vi "运维调试_质控单元.vi"() -> ()   [LabVIEW 2016, in "质控单元.lvlib"]
uses:
  <vilib>/Utility/miscctls.llb/LVPointTypeDef.ctl
  <vilib>/Utility/config.llb/Read Key (I32).vi
  <vilib>/Utility/config.llb/Read Key (Boolean).vi
  <vilib>/Utility/config.llb/Read Key (U32).vi
  <vilib>/Utility/config.llb/Write Key (I32).vi
  <vilib>/Utility/config.llb/Write Key (Boolean).vi
  <vilib>/Utility/config.llb/NI_LVConfig.lvlib
panel:
  out "CODCr状态簇":T1
  out "CODMn状态簇":T1
  out "总氮状态簇":T1
  out "总磷状态簇":T1
  out "氨氮状态簇":T1
  out "总氮柱塞泵故障报警":bool
  out "CODCr柱塞泵故障报警":bool
  out "CODMn柱塞泵故障报警":bool
  out "总磷柱塞泵故障报警":bool
  out "氨氮柱塞泵故障报警":bool
  out "总氮传感器故障报警":bool
  out "总氮传感器状态":bool
  out "总氮流程中断报警":bool
  out "总磷通讯":bool
  out "CODCr质控流程中":bool
  out "CODMn质控流程中":bool
  out "总氮质控流程中":bool caption="总磷质控流程中"
  out "总磷质控流程中":bool caption="总氮质控流程中"
  out "氨氮质控流程中":bool
  out "CODCr通讯":bool
  out "CODMn通讯":bool
  out "总氮通讯":bool
  out "氨氮通讯":bool
  out "CODCr传感器状态":bool
  out "CODCr传感器故障报警":bool
  out "CODMn传感器故障报警":bool
  out "总磷传感器故障报警":bool
  out "氨氮传感器故障报警":bool
  out "CODMn传感器状态":bool
  out "总磷传感器状态":bool
  out "氨氮传感器状态":bool
  out "CODCr流程中断报警":bool
  out "总磷流程中断报警":bool
  out "CODMn流程中断报警":bool
  out "氨氮流程中断报警":bool
  in  "总氮模块选择":bool
  in  "释放串口":bool
  in  "打开串口":bool
  in  "柱塞泵调试":bool
  in  "手动调试":bool
  in  "报警清除":bool
  in  "查看":bool
  in  "停止测量":bool
  in  "加标回收":bool
  in  "平行样测试":bool
  in  "CODCr量程选择":enum32{"H", "L", "AUTO"}(ring)
  in  "CODCr选择":bool
  out "CODCr加标回收率":dbl caption="加标回收率" format="%.2f"
  out "CODCr加标体积":dbl caption="加标体积" format="%.3f"
  out "CODCr母液浓度":dbl caption="加标母液浓度" format="%.2f"
  out "CODCr加标水杯定容体积":dbl caption="加标水杯定容体积" format="%.2f"
  out "CODCr加标后水样浓度":dbl caption="加标后水样浓度" format="%.2f"
  out "CODCr加标前水样浓度":dbl caption="加标前水样浓度" format="%.2f"
  out "CODCr检出限":dbl caption="检出限" format="%.2f"
  out "CODCr量程":dbl caption="量程" format="%.2f"
  out "CODCr状态":u16(ring) caption="状态" items=["待机", "润洗", "进样", "进样完成", "柱塞泵加标", "等待取液", "排液"]
  out "质控流程中":bool
  in  "CODMn量程选择":enum32{"H", "L", "AUTO"}(ring)
  in  "总磷量程选择":enum32{"H", "L", "AUTO"}(ring)=enum."AUTO"
  in  "总氮量程选择":enum32{"H", "L", "AUTO"}(ring)=enum."AUTO"
  in  "氨氮量程选择":enum32{"H", "L", "AUTO"}(ring)=enum."AUTO"
  in  "CODMn选择":bool
  in  "总磷模块选择":bool
  in  "氨氮模块":bool
  in  "背隙补偿步数 3":i32 min=0 max=2000
  in  "背隙补偿步数 2":i32 min=0 max=2000
  in  "背隙补偿步数":i32 min=0 max=2000
  out "总氮加标回收率":dbl caption="加标回收率" format="%.2f"
  out "总氮加标体积":dbl caption="加标体积" format="%.3f"
  out "总氮母液浓度":dbl caption="加标母液浓度" format="%.3f"
  out "总氮加标水杯定容体积":dbl caption="加标水杯定容体积" format="%.2f"
  out "总氮加标后水样浓度":dbl caption="加标后水样浓度" format="%.3f"
  out "总氮加标前水样浓度":dbl caption="加标前水样浓度" format="%.3f"
  out "总氮检出限":dbl caption="检出限" format="%.3f"
  out "总氮量程":dbl caption="量程" format="%.2f"
  out "总氮状态":u16(ring) caption="状态" items=["待机", "润洗", "进样", "进样完成", "柱塞泵加标", "等待取液", "排液"]
  in  "返回":bool
  out "COD平行样测完标志":bool
  out "氨氮总磷平行样测完标志":bool
  out "COD加标回收率":dbl caption="加标回收率" format="%.2f"
  out "COD加标体积":dbl caption="加标体积" format="%.3f"
  out "COD母液浓度":dbl caption="加标母液浓度" format="%.2f"
  out "COD加标水杯定容体积":dbl caption="加标水杯定容体积" format="%.2f"
  out "COD加标后水样浓度":dbl caption="加标后水样浓度" format="%.2f"
  out "COD加标前水样浓度":dbl caption="加标前水样浓度" format="%.2f"
  out "COD检出限":dbl caption="检出限" format="%.2f"
  out "COD量程":dbl caption="量程" format="%.2f"
  out "CODMn状态":u16(ring) caption="状态" items=["待机", "润洗", "进样", "进样完成", "柱塞泵加标", "等待取液", "排液"]
  out "总磷加标回收率":dbl caption="加标回收率" format="%.2f"
  out "总磷加标体积":dbl caption="加标体积" format="%.3f"
  out "总磷母液浓度":dbl caption="加标母液浓度" format="%.3f"
  out "总磷加标水杯定容体积":dbl caption="加标水杯定容体积" format="%.2f"
  out "总磷加标后水样浓度":dbl caption="加标后水样浓度" format="%.3f"
  out "总磷加标前水样浓度":dbl caption="加标前水样浓度" format="%.3f"
  out "总磷检出限":dbl caption="检出限" format="%.3f"
  out "总磷量程":dbl caption="量程" format="%.2f"
  out "总磷状态":u16(ring) caption="状态" items=["待机", "润洗", "进样", "进样完成", "柱塞泵加标", "等待取液", "排液"]
  out "氨氮加标回收率":dbl caption="加标回收率" format="%.2f"
  out "氨氮加标体积":dbl caption="加标体积" format="%.3f"
  out "氨氮母液浓度":dbl caption="加标母液浓度" format="%.3f"
  out "氨氮加标水杯定容体积":dbl caption="加标水杯定容体积" format="%.2f"
  out "氨氮加标后水样浓度":dbl caption="加标后水样浓度" format="%.3f"
  out "氨氮加标前水样浓度":dbl caption="加标前水样浓度" format="%.3f"
  out "氨氮检出限":dbl caption="检出限" format="%.3f"
  out "氨氮量程":dbl caption="量程" format="%.2f"
  out "氨氮状态":u16(ring) caption="状态" items=["待机", "润洗", "进样", "进样完成", "柱塞泵加标", "等待取液", "排液"]
  # "氨氮质控参数"
  # "状态显示区"
  # "参数配置区"
  # "2000步等于1mL\n100步等于0.05mL\n20步等于0.01mL\n2步等于0.001mL\n（初始默认100步）"
  # "柱塞泵调试区"
  # "CODCr质控参数"
  # "%"
  # "mL"
  # "mg/L"
  # "mL"
  # "mg/L"
  # "mg/L"
  # "mg/L"
  # "mg/L"
  # "总氮质控参数"
  # "%"
  # "mL"
  # "mg/L"
  # "mL"
  # "mg/L"
  # "mg/L"
  # "mg/L"
  # "mg/L"
  # "CODMn质控参数"
  # "%"
  # "mL"
  # "mg/L"
  # "mL"
  # "mg/L"
  # "mg/L"
  # "mg/L"
  # "mg/L"
  # "总磷质控参数"
  # "%"
  # "mL"
  # "mg/L"
  # "mL"
  # "mg/L"
  # "mg/L"
  # "mg/L"
  # "mg/L"
  # "%"
  # "mL"
  # "mg/L"
  # "mL"
  # "mg/L"
  # "mg/L"
  # "mg/L"
  # "mg/L"
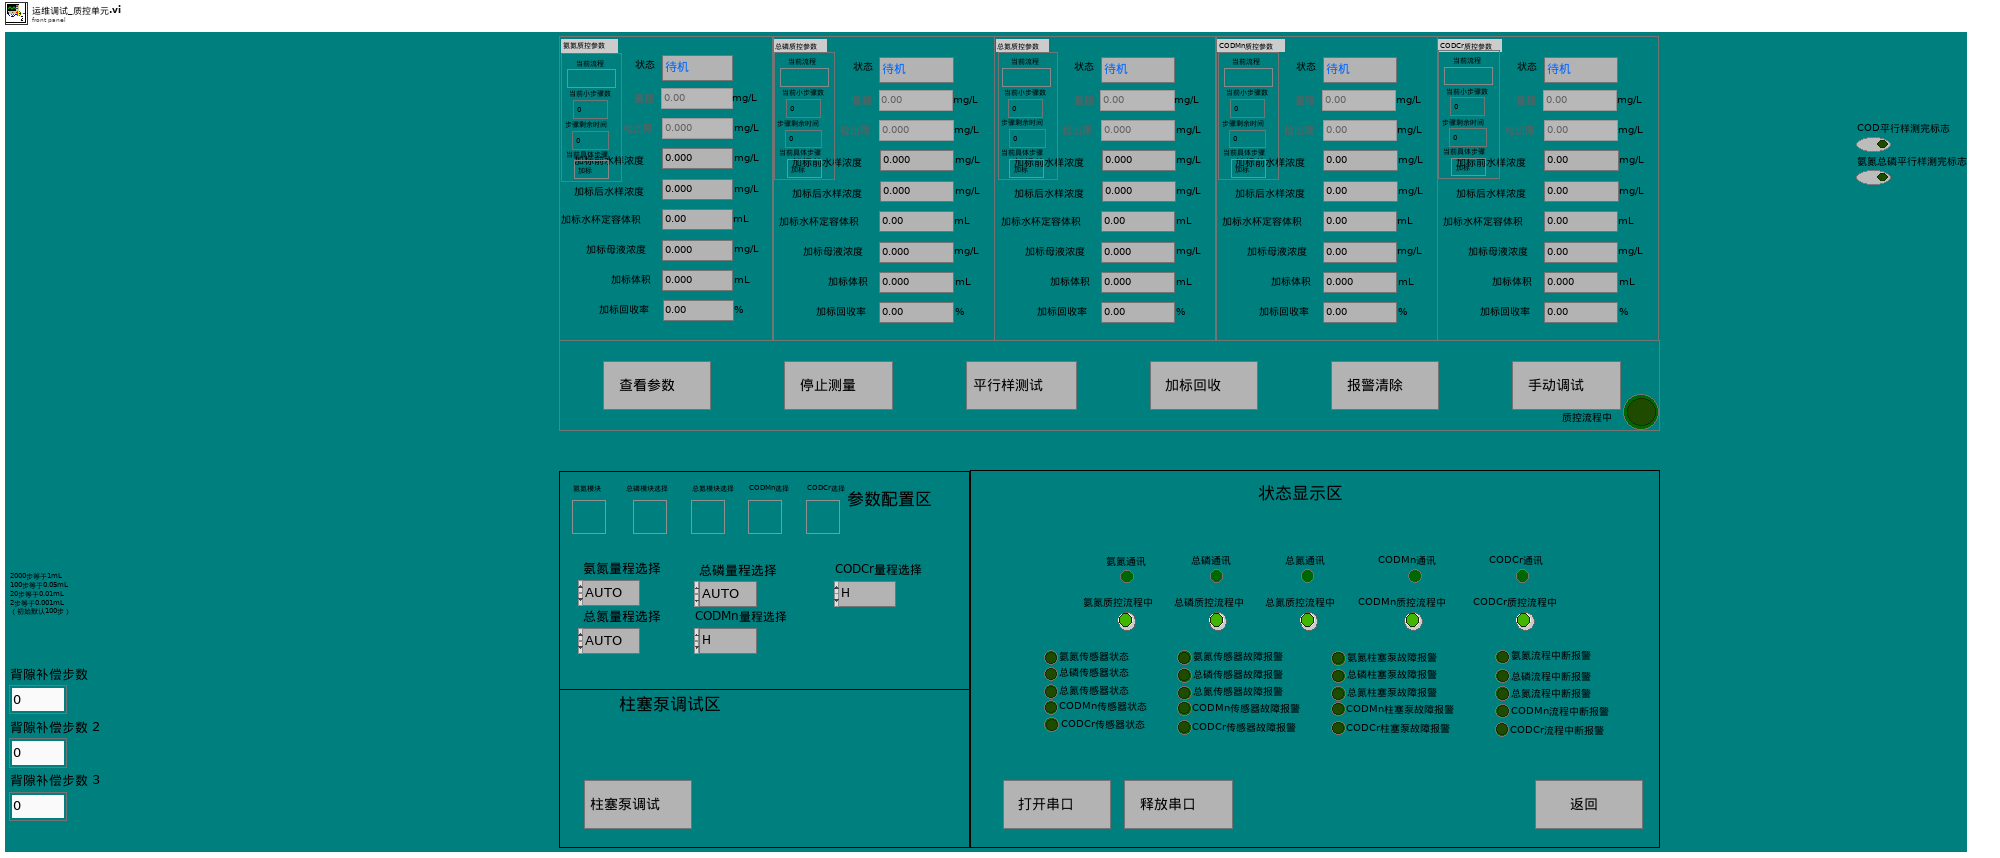
[diagram p1: front panel]
types:
  T1 = cluster{"步骤剩余时间":u16, "当前具体步骤":enum16{"加标", "进样", "排液", "搅拌", "定量"}, " 当前流程":enum16{"", "水样流程", "加标流程", "排液流程"}, "当前小步骤数":i8}
  T2 = typedef "LVPointTypeDef.ctl" = cluster{"Horizontal":i16, "Vertical":i16}
  T3 = typedef "NI_LVConfig.lvlib/Config Data RefNum.ctl" = refnum<k1>
  T4 = cluster{"量程":dbl, "检出限":dbl, "加标前水样浓度":dbl, "加标后水样浓度":dbl, "加标水杯定容体积":dbl, "加标母液浓度":dbl, "加标体积":dbl, "加标回收率":dbl}
  T5 = enum8{"Enabled", "Disabled", "Disabled and Grayed Out"}
  T6 = cluster{"是否启用仪器":bool, "CODMn":cluster{"启动测量模式":cluster{"测量模式":enum16{"水样测量", "标样核查", "加标回收", "平行样", "校零", "校标"}}, "确定按钮":bool}, "启动模块":cluster{"氨氮":bool, "总磷":bool, "总氮":bool, "CODMn":bool, "CODCr":bool}, "常规启动":bool, "直接启动":bool}
  T7 = cluster{"参数启用":cluster{"CODMn":bool, "总磷":bool, "总氮":bool, "氨氮":bool, "CODcr":bool}, "采配水是否启动":bool}
  T8 = cluster{"命令":string, cluster{"starting address":u16, "holding register value":u16}}
  T9 = cluster{"氨氮":bool, "总磷":bool, "总氮":bool, "CODMn":bool, "CODCr":bool}
  T10 = enum32{"Bad", "Idle", "Run top level", "Running"}
  T11 = cluster{"CODMn":bool, "总磷":bool, "总氮":bool, "氨氮":bool, "CODCr":bool}
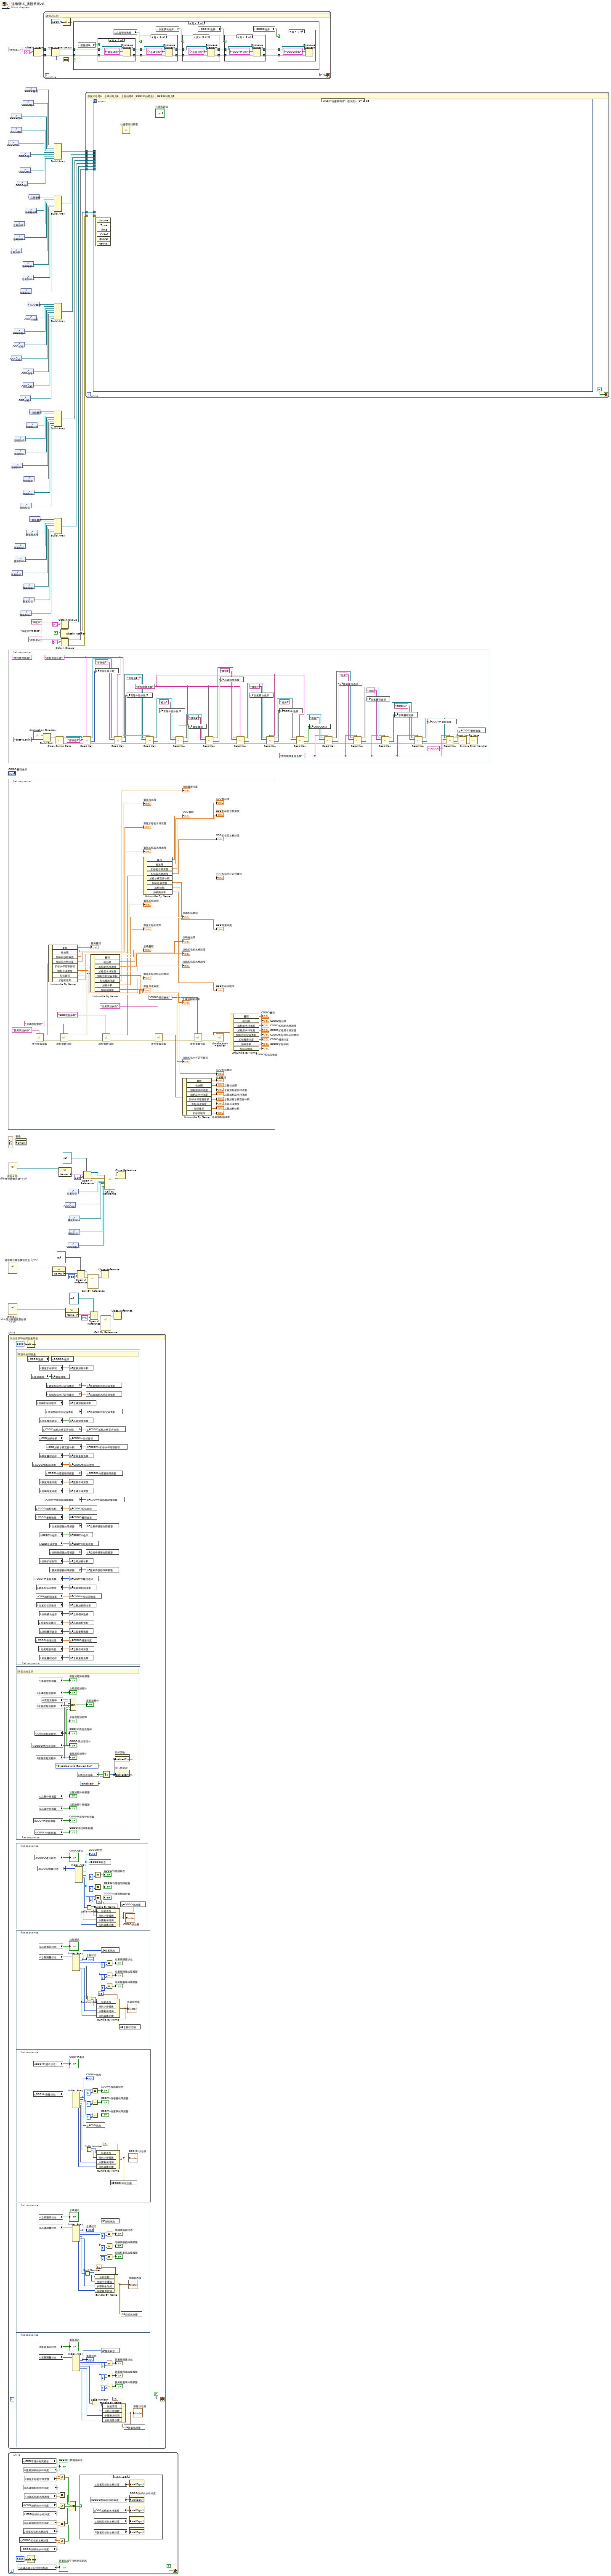
[diagram p0: block diagram]
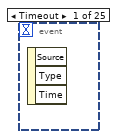
[diagram p9: hidden frame]
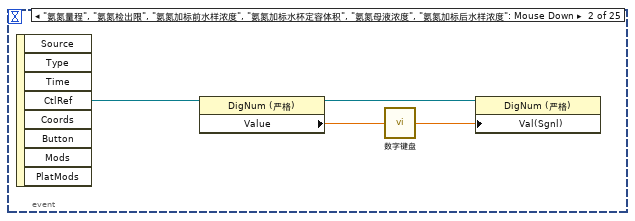
[diagram p10: hidden frame]
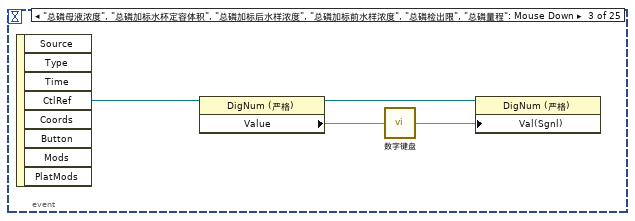
[diagram p11: hidden frame]
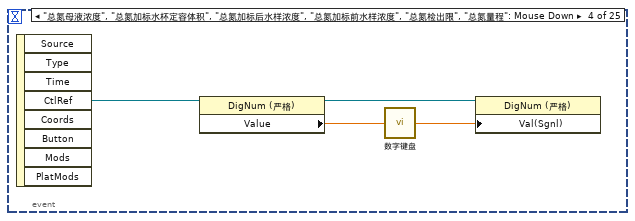
[diagram p12: hidden frame]
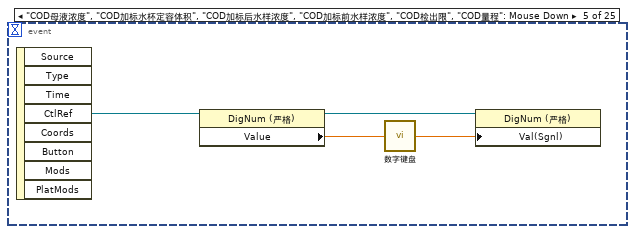
[diagram p13: hidden frame]
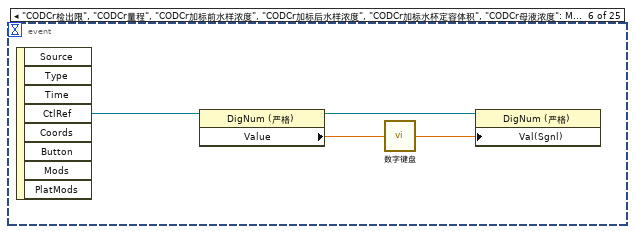
[diagram p14: hidden frame]
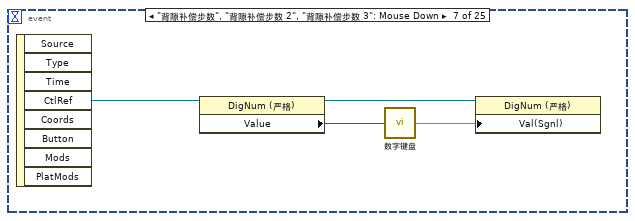
[diagram p15: hidden frame]
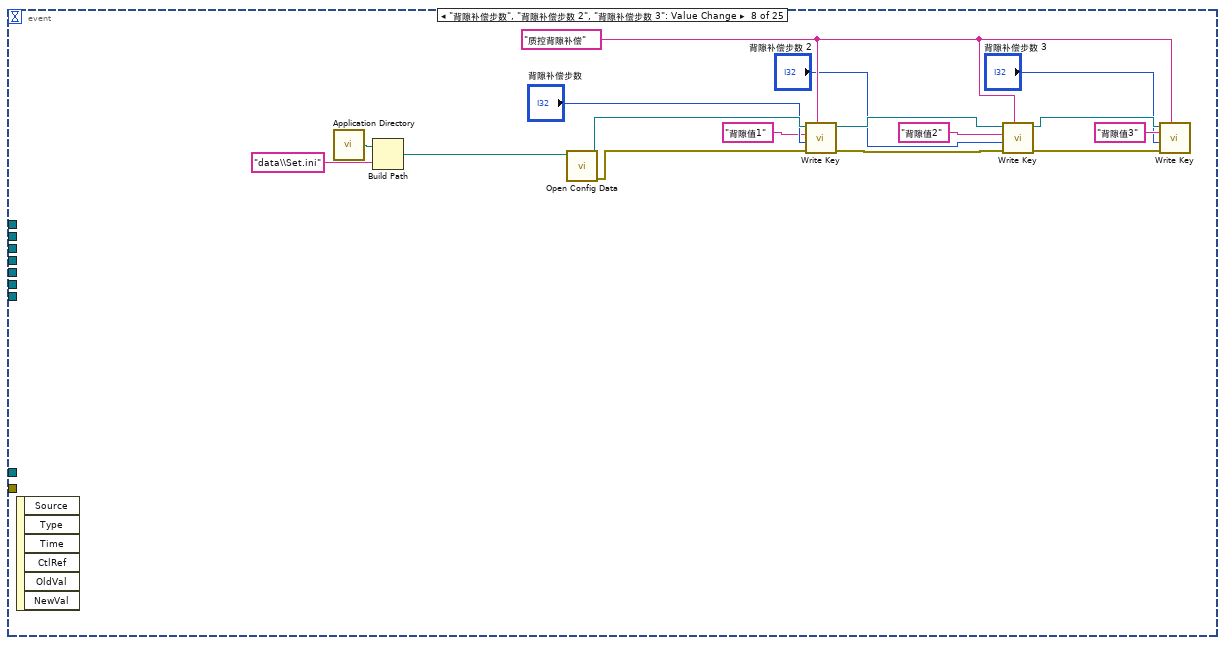
[diagram p16: hidden frame]
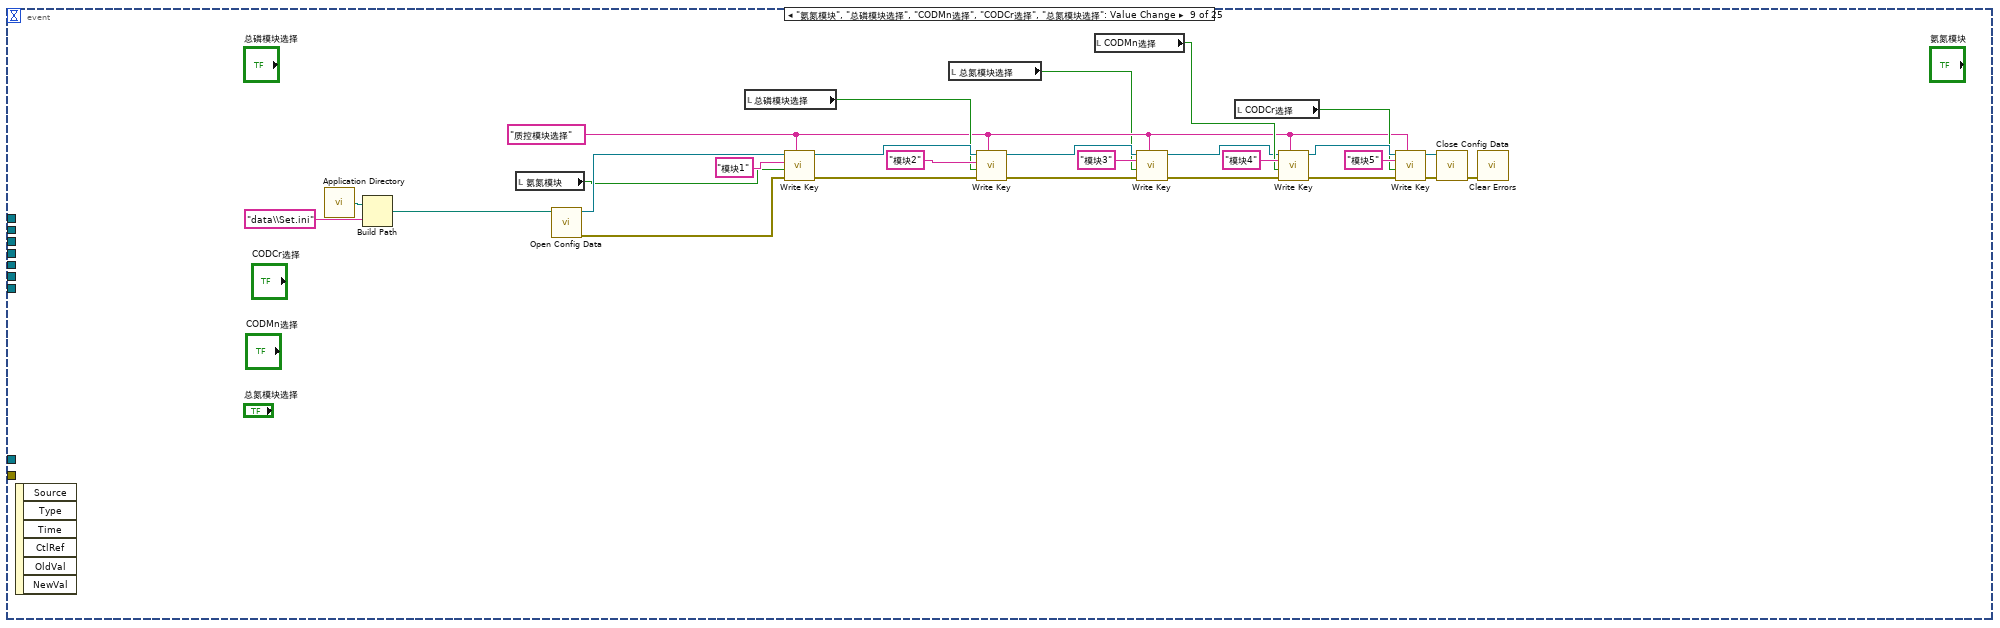
[diagram p17: hidden frame]
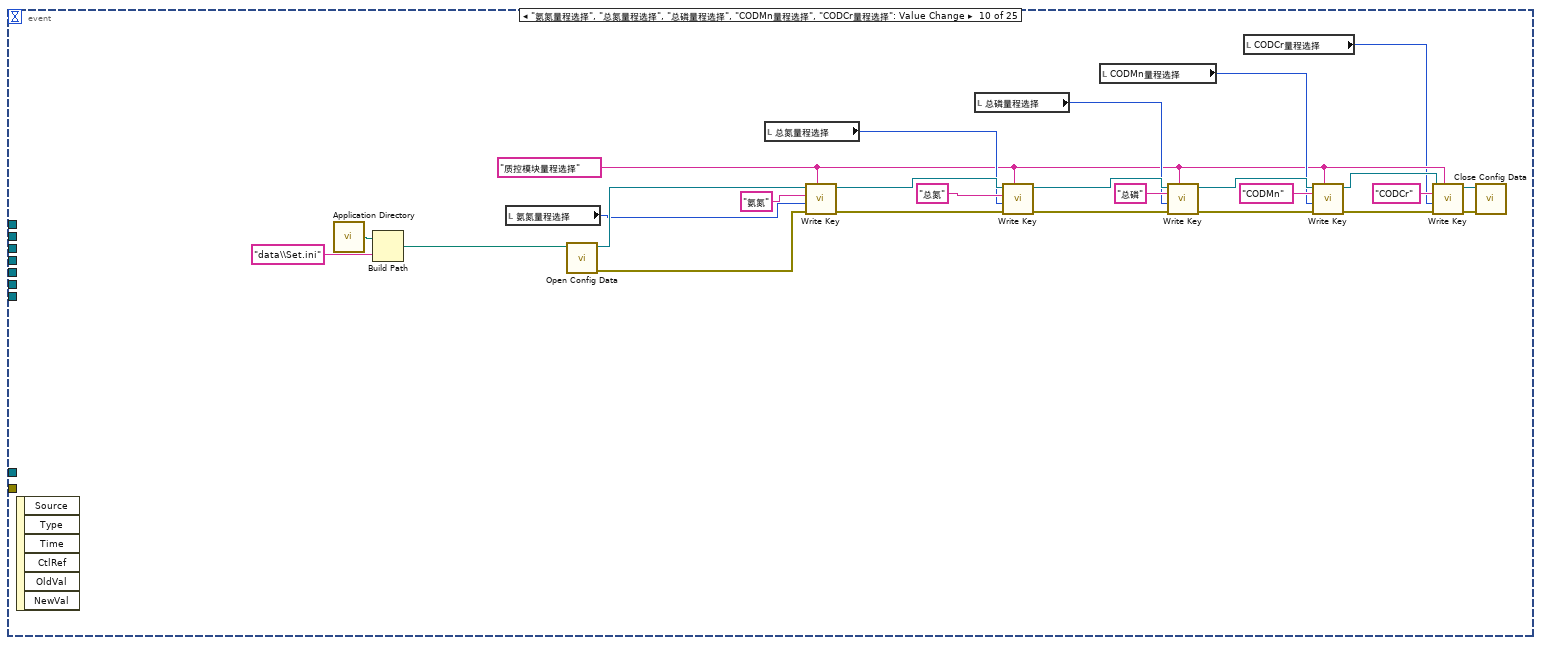
[diagram p18: hidden frame]
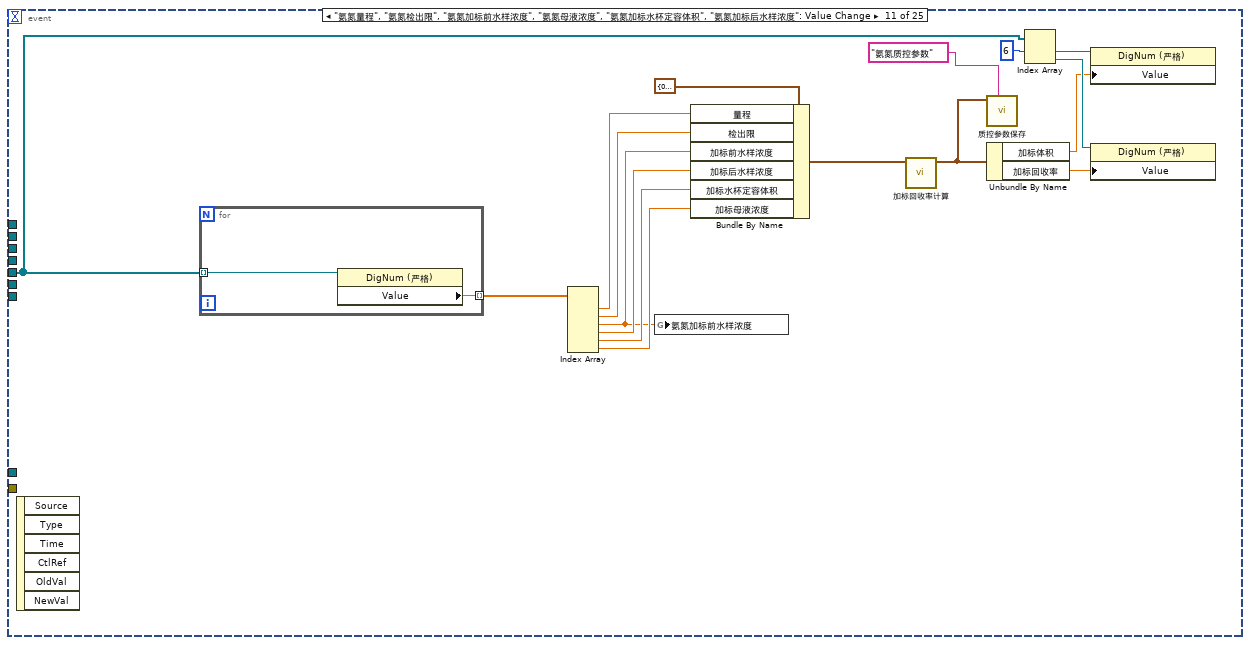
[diagram p19: hidden frame]
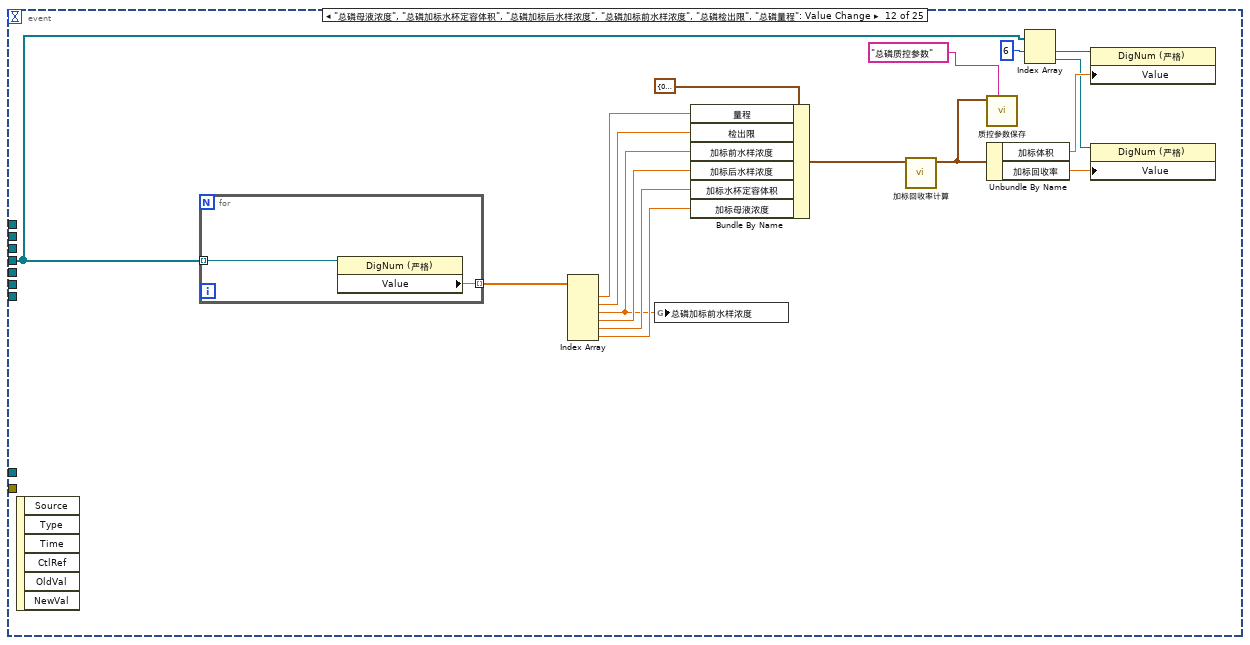
[diagram p20: hidden frame]
diagram:
  n1 = control-ref of="CODCr加标水杯定容体积"() -> (w42:refnum<vi>)
  n2 = flat-sequence {
    frame #0 {
      w110 = "质控模块量程选择" ("section")
      w91 = "质控模块选择" ("section")
      (unwired) "质控线性参数" ("section")
      w144 = "质控背隙补偿" ("section")
      n3 = call <vilib>:"Application Directory.vi"() -> ("Application Directory"=w150:path)
      n4 = Build Path(base path=w150, name or relative path="data\\Set.ini" ("名称或相对路径")) -> (appended path=w148:path)
      n5 = call <vilib>:"Open Config Data.vi"("configuration file path"=w148) -> ("error out"=w146:errorcluster, "refnum"=w147:T3)  [unwired: 8 in, 1 out]
      n6 = call-poly <vilib>:"Read Key.vi"("section"=w144, "error in (no error)"=w146, "key"="背隙值1", "refnum"=w147) -> ("error out"=w141:errorcluster, "value"=w136:i32, "refnum out"=w143:T3)  [unwired: 4 in, 1 out]
      n7 = local write "背隙补偿步数"(w136) -> ()
      n8 = call-poly <vilib>:"Read Key.vi"("section"=w144, "error in (no error)"=w141, "key"="背隙值2", "refnum"=w143) -> ("error out"=w139:errorcluster, "value"=w137:i32, "refnum out"=w140:T3)  [unwired: 4 in, 1 out]
      n9 = local write "背隙补偿步数 2"(w137) -> ()
      n10 = call-poly <vilib>:"Read Key.vi"("section"=w144, "error in (no error)"=w139, "key"="背隙值3", "refnum"=w140) -> ("error out"=w98:errorcluster, "value"=w135:i32, "refnum out"=w99:T3)  [unwired: 4 in, 1 out]
      n11 = local write "背隙补偿步数 3"(w135) -> ()
      n12 = call-poly <vilib>:"Read Key.vi"("section"=w91, "error in (no error)"=w98, "key"="模块1" ("section"), "refnum"=w99) -> ("error out"=w133:errorcluster, "value"=w127:bool, "refnum out"=w134:T3)  [unwired: 4 in, 1 out]
      n13 = local write "氨氮模块"(w127) -> ()
      n14 = call-poly <vilib>:"Read Key.vi"("section"=w91, "error in (no error)"=w133, "key"="模块2" ("section"), "refnum"=w134) -> ("error out"=w95:errorcluster, "value"=w128:bool, "refnum out"=w96:T3)  [unwired: 4 in, 1 out]
      n15 = local write "总磷模块选择"(w128) -> ()
      n16 = call-poly <vilib>:"Read Key.vi"("section"=w91, "error in (no error)"=w95, "key"="模块3" ("section"), "refnum"=w96) -> ("error out"=w93:errorcluster, "value"=w92:bool, "refnum out"=w94:T3)  [unwired: 4 in, 1 out]
      n17 = local write "总氮模块选择"(w92) -> ()
      n18 = call-poly <vilib>:"Read Key.vi"("section"=w91, "error in (no error)"=w93, "key"="模块4" ("section"), "refnum"=w94) -> ("error out"=w104:errorcluster, "value"=w129:bool, "refnum out"=w105:T3)  [unwired: 4 in, 1 out]
      n19 = local write "CODMn选择"(w129) -> ()
      n20 = call-poly <vilib>:"Read Key.vi"("section"=w91, "error in (no error)"=w104, "key"="模块5", "refnum"=w105) -> ("error out"=w101:errorcluster, "value"=w100:bool, "refnum out"=w102:T3)  [unwired: 4 in, 1 out]
      n21 = local write "CODCr选择"(w100) -> ()
      n22 = call-poly <vilib>:"Read Key.vi"("section"=w110, "error in (no error)"=w101, "key"="氨氮" ("section"), "refnum"=w102) -> ("error out"=w125:errorcluster, "value"=w116:u32, "refnum out"=w126:T3)  [unwired: 4 in, 1 out]
      n23 = local write "氨氮量程选择"(w116) -> ()
      n24 = call-poly <vilib>:"Read Key.vi"("section"=w110, "error in (no error)"=w125, "key"="总氮" ("section"), "refnum"=w126) -> ("error out"=w123:errorcluster, "value"=w115:u32, "refnum out"=w124:T3)  [unwired: 4 in, 1 out]
      n25 = local write "总氮量程选择"(w115) -> ()
      n26 = call-poly <vilib>:"Read Key.vi"("section"=w110, "error in (no error)"=w123, "key"="总磷" ("section"), "refnum"=w124) -> ("error out"=w121:errorcluster, "value"=w114:u32, "refnum out"=w122:T3)  [unwired: 4 in, 1 out]
      n27 = local write "总磷量程选择"(w114) -> ()
      n28 = call-poly <vilib>:"Read Key.vi"("section"=w110, "error in (no error)"=w121, "key"="CODMn" ("section"), "refnum"=w122) -> ("error out"=w111:errorcluster, "value"=w113:u32, "refnum out"=w112:T3)  [unwired: 4 in, 1 out]
      n29 = local write "CODMn量程选择"(w113) -> ()
      n30 = call-poly <vilib>:"Read Key.vi"("section"=w110, "error in (no error)"=w111, "key"="CODCr" ("section"), "refnum"=w112) -> ("error out"=w107:errorcluster, "value"=w108:u32, "refnum out"=w106:T3)  [unwired: 4 in, 1 out]
      n31 = local write "CODCr量程选择"(w108) -> ()
      n32 = call <vilib>:"Close Config Data.vi"("error in (no error)"=w107, "refnum"=w106) -> ("error out"=w90:errorcluster)  [unwired: 8 in, 1 out]
      n33 = call <vilib>:"Simple Error Handler.vi"("error in (no error)"=w90) -> ()  [unwired: 4 in, 5 out]
    }
  }
  n34 = flat-sequence {
    frame #0 {
      n35 = call "质控参数读取.vi"("section"="氨氮质控参数") -> ("error out"=w185:errorcluster, "参数"=w204:T4)  [unwired: 9 in]
      n36 = Unbundle By Name(w204) -> ("量程"=→"氨氮量程":dbl, "检出限"=→"氨氮检出限":dbl, "加标前水样浓度"=→"氨氮加标前水样浓度":dbl, "加标后水样浓度"=→"氨氮加标后水样浓度":dbl, "加标水杯定容体积"=→"氨氮加标水杯定容体积":dbl, "加标母液浓度"=→"氨氮母液浓度":dbl, "加标体积"=→"氨氮加标体积":dbl, "加标回收率"=→"氨氮加标回收率":dbl)
      n37 = call "质控参数读取.vi"("section"="总磷质控参数", "error in (no error)"=w185) -> ("error out"=w182:errorcluster, "参数"=w194:T4)  [unwired: 8 in]
      n38 = Unbundle By Name(w194) -> ("量程"=→"总磷量程":dbl, "检出限"=→"总磷检出限":dbl, "加标前水样浓度"=→"总磷加标前水样浓度":dbl, "加标后水样浓度"=→"总磷加标后水样浓度":dbl, "加标水杯定容体积"=→"总磷加标水杯定容体积":dbl, "加标母液浓度"=→"总磷母液浓度":dbl, "加标体积"=→"总磷加标体积":dbl, "加标回收率"=→"总磷加标回收率":dbl)
      n39 = call "质控参数读取.vi"("section"="COD质控参数", "error in (no error)"=w182) -> ("error out"=w172:errorcluster, "参数"=w184:T4)  [unwired: 8 in]
      n40 = Unbundle By Name(w184) -> ("量程"=→"COD量程":dbl, "检出限"=→"COD检出限":dbl, "加标前水样浓度"=→"COD加标前水样浓度":dbl, "加标后水样浓度"=→"COD加标后水样浓度":dbl, "加标水杯定容体积"=→"COD加标水杯定容体积":dbl, "加标母液浓度"=→"COD母液浓度":dbl, "加标体积"=→"COD加标体积":dbl, "加标回收率"=→"COD加标回收率":dbl)
      n41 = call "质控参数读取.vi"("section"="总氮质控参数", "error in (no error)"=w172) -> ("error out"=w160:errorcluster, "参数"=w171:T4)  [unwired: 8 in]
      n42 = Unbundle By Name(w171) -> ("量程"=→"总氮量程":dbl, "检出限"=→"总氮检出限":dbl, "加标前水样浓度"=→"总氮加标前水样浓度":dbl, "加标后水样浓度"=→"总氮加标后水样浓度":dbl, "加标水杯定容体积"=→"总氮加标水杯定容体积":dbl, "加标母液浓度"=→"总氮母液浓度":dbl, "加标体积"=→"总氮加标体积":dbl, "加标回收率"=→"总氮加标回收率":dbl)
      n43 = call "质控参数读取.vi"("section"="CODCr质控参数", "error in (no error)"=w160) -> ("error out"=w151:errorcluster, "参数"=w161:T4)  [unwired: 8 in]
      n44 = call <vilib>:"Simple Error Handler.vi"("error in (no error)"=w151) -> ()  [unwired: 4 in, 5 out]
      n45 = Unbundle By Name(w161) -> ("量程"=→"CODCr量程":dbl, "检出限"=→"CODCr检出限":dbl, "加标前水样浓度"=→"CODCr加标前水样浓度":dbl, "加标后水样浓度"=→"CODCr加标后水样浓度":dbl, "加标水杯定容体积"=→"CODCr加标水杯定容体积":dbl, "加标母液浓度"=→"CODCr母液浓度":dbl, "加标体积"=→"CODCr加标体积":dbl, "加标回收率"=→"CODCr加标回收率":dbl)
    }
  }
  n46 = vi-ref "质控单元.lvlib:质控数据存储(子VI).vi"() -> (w17:refnum<vi>)
  n47 = vi-ref "通信并与其他模块交互 (子VI).vi"() -> (w30:refnum<vi>)
  n48 = vi-ref "质控单元.lvlib:质控报警信息存储 (子VI).vi"() -> (w25:refnum<vi>)
  n49 = while {
    stop <- FALSE stop-if-true
    # "状态显示和全局变量赋值"
    n50 = flat-sequence {
      frame #0 {
        # "赋值给全局变量"
        n51 = local read "CODCr选择"() -> (w341:bool)
        n52 = local read "氨氮模块"() -> (w340:bool)
        n53 = local read "CODCr加标回收率"() -> (w323:dbl)
        n54 = local read "CODMn量程选择"() -> (w347:enum32{"H", "L", "AUTO"})
        n55 = local read "CODCr加标体积"() -> (w334:dbl)
        n56 = local read "CODCr量程选择"() -> (w348:enum32{"H", "L", "AUTO"})
        n57 = local read "CODCr母液浓度"() -> (w324:dbl)
        n58 = local read "COD加标回收率"() -> (w322:dbl)
        n59 = local read "总磷加标回收率"() -> (w320:dbl)
        n60 = local read "氨氮加标回收率"() -> (w319:dbl)
        n61 = local read "总氮加标回收率"() -> (w321:dbl)
        n62 = local read "总氮加标体积"() -> (w336:dbl)
        n63 = local read "总氮母液浓度"() -> (w326:dbl)
        n64 = local read "COD加标体积"() -> (w335:dbl)
        n65 = local read "COD母液浓度"() -> (w325:dbl)
        n66 = local read "氨氮加标体积"() -> (w338:dbl)
        n67 = local read "总氮模块选择"() -> (w343:bool)
        n68 = local read "氨氮量程选择"() -> (w346:enum32{"H", "L", "AUTO"})
        n69 = local read "氨氮母液浓度"() -> (w328:dbl)
        n70 = local read "总磷母液浓度"() -> (w327:dbl)
        n71 = local read "总磷加标体积"() -> (w337:dbl)
        n72 = local read "总磷模块选择"() -> (w339:bool)
        n73 = local read "总磷量程选择"() -> (w344:enum32{"H", "L", "AUTO"})
        n74 = local read "总氮量程选择"() -> (w345:enum32{"H", "L", "AUTO"})
        n75 = local read "CODMn选择"() -> (w342:bool)
        n76 = local read "CODCr加标水杯定容体积"() -> (w333:dbl)
        n77 = local read "CODMn传感器故障报警"() -> (w315:bool)
        n78 = local read "总氮加标水杯定容体积"() -> (w331:dbl)
        n79 = local read "CODCr传感器故障报警"() -> (w314:bool)
        n80 = local read "COD加标水杯定容体积"() -> (w332:dbl)
        n81 = local read "氨氮加标水杯定容体积"() -> (w329:dbl)
        n82 = local read "总磷加标水杯定容体积"() -> (w330:dbl)
        n83 = local read "总氮传感器故障报警"() -> (w316:bool)
        n84 = local read "总磷传感器故障报警"() -> (w317:bool)
        n85 = local read "氨氮传感器故障报警"() -> (w318:bool)
        n86 = global write "断电保存全局.vi" "CODCr选择"(w341) -> ()
        n87 = global write "断电保存全局.vi" "氨氮模块"(w340) -> ()
        n88 = global write "加标回收状态全局变量.vi" "氨氮加标体积"(w338) -> ()
        n89 = global write "加标回收状态全局变量.vi" "总磷加标回收率"(w320) -> ()
        n90 = global write "断电保存全局.vi" "总氮模块选择"(w343) -> ()
        n91 = global write "加标回收状态全局变量.vi" "CODMn加标体积"(w335) -> ()
        n92 = global write "断电保存全局.vi" "氨氮量程选择"(w346) -> ()
        n93 = global write "加标回收状态全局变量.vi" "CODCr加标回收率"(w323) -> ()
        n94 = global write "加标回收状态全局变量.vi" "氨氮母液浓度"(w328) -> ()
        n95 = global write "加标回收状态全局变量.vi" "总磷母液浓度"(w327) -> ()
        n96 = global write "加标回收状态全局变量.vi" "CODCr加标体积"(w334) -> ()
        n97 = global write "断电保存全局.vi" "CODCr量程选择"(w348) -> ()
        n98 = global write "断电保存全局.vi" "CODMn选择"(w342) -> ()
        n99 = global write "加标回收状态全局变量.vi" "CODMn母液浓度"(w325) -> ()
        n100 = global write "加标回收状态全局变量.vi" "总磷加标体积"(w337) -> ()
        n101 = global write "断电保存全局.vi" "CODMn量程选择"(w347) -> ()
        n102 = global write "加标回收状态全局变量.vi" "氨氮加标回收率"(w319) -> ()
        n103 = global write "加标回收状态全局变量.vi" "CODMn加标回收率"(w322) -> ()
        n104 = global write "加标回收状态全局变量.vi" "总氮加标回收率"(w321) -> ()
        n105 = global write "断电保存全局.vi" "总磷模块选择"(w339) -> ()
        n106 = global write "加标回收状态全局变量.vi" "总氮加标体积"(w336) -> ()
        n107 = global write "断电保存全局.vi" "总磷量程选择"(w344) -> ()
        n108 = global write "加标回收状态全局变量.vi" "CODCr母液浓度"(w324) -> ()
        n109 = global write "加标回收状态全局变量.vi" "总氮母液浓度"(w326) -> ()
        n110 = global write "断电保存全局.vi" "总氮量程选择"(w345) -> ()
        n111 = global write "加标回收状态全局变量.vi" "氨氮加标水杯定容体积"(w329) -> ()
        n112 = global write "加标回收状态全局变量.vi" "总磷加标水杯定容体积"(w330) -> ()
        n113 = global write "加标回收状态全局变量.vi" "总氮加标水杯定容体积"(w331) -> ()
        n114 = global write "加标回收状态全局变量.vi" "CODCr加标水杯定容体积"(w333) -> ()
        n115 = global write "加标回收状态全局变量.vi" "CODMn加标水杯定容体积"(w332) -> ()
        n116 = global write "质控中断报警全局.vi" "CODCr传感器故障报警"(w314) -> ()
        n117 = global write "质控中断报警全局.vi" "CODMn传感器故障报警"(w315) -> ()
        n118 = global write "质控中断报警全局.vi" "总氮传感器故障报警"(w316) -> ()
        n119 = global write "质控中断报警全局.vi" "总磷传感器故障报警"(w317) -> ()
        n120 = global write "质控中断报警全局.vi" "氨氮传感器故障报警"(w318) -> ()
      }
    }
    n121 = flat-sequence {
      frame #0 {
        # "界面状态显示"
        n122 = global read "质控测完标志全局 1.vi" "CODCr质控流程中"() -> (w304:bool)
        "CODCr质控流程中" <- w304
        n123 = global read "质控中断报警全局.vi" "CODMn中断报警"() -> (→"CODMn流程中断报警":bool)
        n124 = global read "质控测完标志全局 1.vi" "COD质控流程中"() -> (w303:bool)
        "CODMn质控流程中" <- w303
        n125 = global read "质控中断报警全局.vi" "CODCr中断报警"() -> (→"CODCr流程中断报警":bool)
        n126 = global read "质控测完标志全局 1.vi" "总磷质控流程中"() -> (w302:bool)
        "总磷质控流程中" <- w302
        n127 = global read "质控测完标志全局 1.vi" "总氮质控流程中"() -> (w305:bool)
        "总氮质控流程中" <- w305
        n128 = global read "质控测完标志全局 1.vi" "氨氮质控流程中"() -> (w301:bool)
        "氨氮质控流程中" <- w301
        n129 = global read "质控中断报警全局.vi" "氨氮中断报警"() -> (→"氨氮流程中断报警":bool)
        n130 = global read "质控中断报警全局.vi" "总氮中断报警"() -> (→"总氮流程中断报警":bool)
        n131 = global read "质控中断报警全局.vi" "总磷中断报警"() -> (→"总磷流程中断报警":bool)
        n132 = global read "质控测完标志全局 1.vi" "质控流程中"() -> (w299:bool)
        n133 = Compound Arithmetic op=OR ("复合运算")(w299, w301, w302, w305, w303, w304) -> (→"质控流程中":bool)
        n134 = global read "质控测完标志全局 1.vi" "质控流程中"() -> (w309:bool)
        n135 = Select(t=T5."Disabled and Grayed Out" ("禁用"), s=w309, f=T5."Enabled") -> (s? t:f=w298:T5)
        n136 = property on="加标回收" class="Bool"("DisabledEnum"=w298) -> ()  [unwired: 2 in, 2 out]
        n137 = property on="平行样测试" class="Bool"("DisabledEnum"=w298) -> ()  [unwired: 2 in, 2 out]
      }
    }
    n138 = flat-sequence {
      frame #0 {
        n139 = global read "质控内部交互全局.vi" "CODCr通讯状态"() -> (→"CODCr通讯":bool)
        n140 = global read "质控内部交互全局.vi" "CODCr测量状态"() -> (w242:u16[])
        n141 = Index Array(array=w242) -> (element #1=w243:u16, element #2=w238:u16, element #3=w234:u16, element #4=w232:u16, element #5=w229:u16, element #6=w228:u16)  [unwired: 6 in]
        "CODCr状态" <- w243
        n142 = Split Number(x=w232) -> (hi(x)=w231:u8, lo(x)=w230:u8)
        n143 = global write "加标回收状态全局变量.vi" "CODCr状态"(w243) -> ()
        n144 = Equal?(x=w238, y=u16 1) -> (x = y?=→"CODCr传感器状态":bool)
        n145 = Equal?(x=w234, y=u16 1) -> (x = y?=→"CODCr传感器故障报警":bool)
        n146 = Equal?(x=w234, y=u16 2) -> (x = y?=→"CODCr柱塞泵故障报警":bool)
        n147 = Bundle By Name(cluster=T1 {"步骤剩余时间"=0, "当前具体步骤"=enum."加标", " 当前流程"=enum."", "当前小步骤数"=0} ("氨氮状态簇"), "当前流程"=w231, "当前小步骤数"=w230, "步骤剩余时间"=w229, "当前具体步骤"=w228) -> (w226:T1)
        "CODCr状态簇" <- w226
        n148 = global write "加标回收状态全局变量.vi" "CODCr状态簇"(w226) -> ()
      }
    }
    n149 = flat-sequence {
      frame #0 {
        n150 = global read "质控内部交互全局.vi" "总氮通讯状态"() -> (→"总氮通讯":bool)
        n151 = global read "质控内部交互全局.vi" "总氮测量状态"() -> (w222:u16[])
        n152 = Index Array(array=w222) -> (element #1=w221:u16, element #2=w224:u16, element #3=w216:u16, element #4=w212:u16, element #5=w210:u16, element #6=w211:u16)  [unwired: 6 in]
        "总氮状态" <- w221
        n153 = Split Number(x=w212) -> (hi(x)=w214:u8, lo(x)=w213:u8)
        n154 = Bundle By Name(cluster=T1 {"步骤剩余时间"=0, "当前具体步骤"=enum."加标", " 当前流程"=enum."", "当前小步骤数"=0} ("氨氮状态簇"), "当前流程"=w214, "当前小步骤数"=w213, "步骤剩余时间"=w210, "当前具体步骤"=w211) -> (w208:T1)
        "总氮状态簇" <- w208
        n155 = global write "加标回收状态全局变量.vi" "总氮状态"(w221) -> ()
        n156 = Equal?(x=w224, y=u16 1) -> (x = y?=→"总氮传感器状态":bool)
        n157 = Equal?(x=w216, y=u16 1) -> (x = y?=→"总氮传感器故障报警":bool)
        n158 = Equal?(x=w216, y=u16 2) -> (x = y?=→"总氮柱塞泵故障报警":bool)
        n159 = global write "加标回收状态全局变量.vi" "总氮状态簇"(w208) -> ()
      }
    }
    n160 = flat-sequence {
      frame #0 {
        n161 = global read "质控内部交互全局.vi" "CODMn通讯状态"() -> (→"CODMn通讯":bool)
        n162 = global read "质控内部交互全局.vi" "CODMn测量状态"() -> (w258:u16[])
        n163 = Index Array(array=w258) -> (element #1=w261:u16, element #2=w259:u16, element #3=w252:u16, element #4=w248:u16, element #5=w246:u16, element #6=w247:u16)  [unwired: 6 in]
        "CODMn状态" <- w261
        n164 = Split Number(x=w248) -> (hi(x)=w250:u8, lo(x)=w249:u8)
        n165 = global write "加标回收状态全局变量.vi" "COD状态"(w261) -> ()
        n166 = Equal?(x=w259, y=u16 1) -> (x = y?=→"CODMn传感器状态":bool)
        n167 = Equal?(x=w252, y=u16 1) -> (x = y?=→"CODMn传感器故障报警":bool)
        n168 = Equal?(x=w252, y=u16 2) -> (x = y?=→"CODMn柱塞泵故障报警":bool)
        n169 = Bundle By Name(cluster=T1 {"步骤剩余时间"=0, "当前具体步骤"=enum."加标", " 当前流程"=enum."", "当前小步骤数"=0} ("氨氮状态簇"), "当前流程"=w250, "当前小步骤数"=w249, "步骤剩余时间"=w246, "当前具体步骤"=w247) -> (w244:T1)
        "CODMn状态簇" <- w244
        n170 = global write "加标回收状态全局变量.vi" "CODMn状态簇"(w244) -> ()
      }
    }
    n171 = flat-sequence {
      frame #0 {
        n172 = global read "质控内部交互全局.vi" "总磷通讯状态"() -> (→"总磷通讯":bool)
        n173 = global read "质控内部交互全局.vi" "总磷测量状态"() -> (w276:u16[])
        n174 = Index Array(array=w276) -> (element #1=w277:u16, element #2=w278:u16, element #3=w270:u16, element #4=w266:u16, element #5=w264:u16, element #6=w265:u16)  [unwired: 6 in]
        "总磷状态" <- w277
        n175 = Split Number(x=w266) -> (hi(x)=w268:u8, lo(x)=w267:u8)
        n176 = Bundle By Name(cluster=T1 {"步骤剩余时间"=0, "当前具体步骤"=enum."加标", " 当前流程"=enum."", "当前小步骤数"=0} ("氨氮状态簇"), "当前流程"=w268, "当前小步骤数"=w267, "步骤剩余时间"=w264, "当前具体步骤"=w265) -> (w262:T1)
        "总磷状态簇" <- w262
        n177 = global write "加标回收状态全局变量.vi" "总磷状态"(w277) -> ()
        n178 = Equal?(x=w278, y=u16 1) -> (x = y?=→"总磷传感器状态":bool)
        n179 = Equal?(x=w270, y=u16 1) -> (x = y?=→"总磷传感器故障报警":bool)
        n180 = Equal?(x=w270, y=u16 2) -> (x = y?=→"总磷柱塞泵故障报警":bool)
        n181 = global write "加标回收状态全局变量.vi" "总磷状态簇"(w262) -> ()
      }
    }
    n182 = flat-sequence {
      frame #0 {
        n183 = global read "质控内部交互全局.vi" "氨氮通讯状态"() -> (→"氨氮通讯":bool)
        n184 = global read "质控内部交互全局.vi" "氨氮测量状态"() -> (w294:u16[])
        n185 = Index Array(array=w294) -> (element #1=w295:u16, element #2=w297:u16, element #3=w288:u16, element #4=w284:u16, element #5=w282:u16, element #6=w283:u16)  [unwired: 6 in]
        "氨氮状态" <- w295
        n186 = Split Number(x=w284) -> (hi(x)=w286:u8, lo(x)=w285:u8)
        n187 = global write "加标回收状态全局变量.vi" "氨氮状态"(w295) -> ()
        n188 = Bundle By Name(cluster=T1 {"步骤剩余时间"=0, "当前具体步骤"=enum."加标", " 当前流程"=enum."", "当前小步骤数"=0} ("氨氮状态簇"), "当前流程"=w286, "当前小步骤数"=w285, "步骤剩余时间"=w282, "当前具体步骤"=w283) -> (w280:T1)
        "氨氮状态簇" <- w280
        n189 = Equal?(x=w297, y=u16 1) -> (x = y?=→"氨氮传感器状态":bool)
        n190 = Equal?(x=w288, y=u16 1) -> (x = y?=→"氨氮传感器故障报警":bool)
        n191 = Equal?(x=w288, y=u16 2) -> (x = y?=→"氨氮柱塞泵故障报警":bool)
        n192 = global write "加标回收状态全局变量.vi" "氨氮状态簇"(w280) -> ()
      }
    }
    n193 = Wait (ms)(milliseconds to wait=u32 1000 ("等待时间（毫秒）")) -> ()  [unwired: 1 out]
  }
  n194 = while {
    stop <- FALSE stop-if-true
    n195 = global read "质控测完标志全局 1.vi" "总磷总氮平行样测完标志"() -> (→"氨氮总磷平行样测完标志":bool)
    n196 = global read "水样浓度全局.vi" "CODCr加标前水样浓度"() -> (w351:dbl)
    n197 = local read "CODCr加标前水样浓度"() -> (w350:dbl)
    n198 = global read "质控测完标志全局 1.vi" "COD平行样测完标志"() -> (→"COD平行样测完标志":bool)
    n199 = global read "水样浓度全局.vi" "COD加标前水样浓度"() -> (w362:dbl)
    n200 = local read "总氮加标前水样浓度"() -> (w354:dbl)
    n201 = global read "水样浓度全局.vi" "氨氮加标前水样浓度"() -> (w366:dbl)
    n202 = global read "水样浓度全局.vi" "总磷加标前水样浓度"() -> (w364:dbl)
    n203 = local read "COD加标前水样浓度"() -> (w361:dbl)
    n204 = global read "水样浓度全局.vi" "总氮加标前水样浓度"() -> (w353:dbl)
    n205 = local read "氨氮加标前水样浓度"() -> (w365:dbl)
    n206 = local read "总磷加标前水样浓度"() -> (w363:dbl)
    n207 = Wait (ms)(milliseconds to wait=u32 1000 ("等待时间（毫秒）")) -> ()  [unwired: 1 out]
    n208 = Not Equal?(x=w366, y=w365) -> (x != y?=w360:bool)
    n209 = Not Equal?(x=w364, y=w363) -> (x != y?=w358:bool)
    n210 = Not Equal?(x=w362, y=w361) -> (x != y?=w357:bool)
    n211 = Not Equal?(x=w353, y=w354) -> (x != y?=w352:bool)
    n212 = Not Equal?(x=w351, y=w350) -> (x != y?=w349:bool)
    n213 = Compound Arithmetic op=OR ("复合运算")(w360, w358, w357, w352, w349) -> (w359:bool)
    n214 = case shown="真" w359 {
      frame False {
      }
      frame True {
        n215 = global read "水样浓度全局.vi" "CODCr加标前水样浓度"() -> (w369:dbl)
        n216 = global read "水样浓度全局.vi" "COD加标前水样浓度"() -> (w371:dbl)
        n217 = global read "水样浓度全局.vi" "总氮加标前水样浓度"() -> (w370:dbl)
        n218 = global read "水样浓度全局.vi" "总磷加标前水样浓度"() -> (w372:dbl)
        n219 = global read "水样浓度全局.vi" "氨氮加标前水样浓度"() -> (w373:dbl)
        n220 = property on="总氮加标前水样浓度" class="DigNum (严格)"("Val(Sgnl)"=w370) -> ()  [unwired: 2 in, 2 out]
        n221 = property on="CODCr加标前水样浓度" class="DigNum (严格)"("Val(Sgnl)"=w369) -> ()  [unwired: 2 in, 2 out]
        n222 = property on="COD加标前水样浓度" class="DigNum (严格)"("Val(Sgnl)"=w371) -> ()  [unwired: 2 in, 2 out]
        n223 = property on="总磷加标前水样浓度" class="DigNum (严格)"("Val(Sgnl)"=w372) -> ()  [unwired: 2 in, 2 out]
        n224 = property on="氨氮加标前水样浓度" class="DigNum (严格)"("Val(Sgnl)"=w373) -> ()  [unwired: 2 in, 2 out]
      }
    }
  }
  n225 = control-ref of="CODCr加标前水样浓度"() -> (w44:refnum<vi>)
  n226 = control-ref of="CODCr加标后水样浓度"() -> (w43:refnum<vi>)
  n227 = control-ref of="总氮加标水杯定容体积"() -> (w51:refnum<vi>)
  n228 = control-ref of="COD加标水杯定容体积"() -> (w66:refnum<vi>)
  n229 = control-ref of="总磷加标水杯定容体积"() -> (w75:refnum<vi>)
  n230 = control-ref of="氨氮加标水杯定容体积"() -> (w85:refnum<vi>)
  n231 = control-ref of="总氮加标前水样浓度"() -> (w53:refnum<vi>)
  n232 = control-ref of="总氮加标后水样浓度"() -> (w52:refnum<vi>)
  n233 = control-ref of="COD加标前水样浓度"() -> (w68:refnum<vi>)
  n234 = control-ref of="COD加标后水样浓度"() -> (w67:refnum<vi>)
  n235 = control-ref of="总磷加标前水样浓度"() -> (w77:refnum<vi>)
  n236 = control-ref of="总磷加标后水样浓度"() -> (w76:refnum<vi>)
  n237 = control-ref of="氨氮加标前水样浓度"() -> (w86:refnum<vi>)
  n238 = control-ref of="氨氮加标后水样浓度"() -> (w82:refnum<vi>)
  n239 = property on="窗格" class="Pane"("Origin"=T2 {"Horizontal"=0, "Vertical"=0} ("原点")) -> ()  [unwired: 2 in, 2 out]
  n240 = control-ref of="CODCr加标回收率"() -> (w39:refnum<vi>)
  n241 = control-ref of="CODCr母液浓度"() -> (w41:refnum<vi>)
  n242 = control-ref of="CODCr加标体积"() -> (w40:refnum<vi>)
  n243 = control-ref of="COD加标回收率"() -> (w63:refnum<vi>)
  n244 = control-ref of="总氮加标回收率"() -> (w48:refnum<vi>)
  n245 = control-ref of="总磷加标回收率"() -> (w73:refnum<vi>)
  n246 = control-ref of="氨氮加标回收率"() -> (w80:refnum<vi>)
  n247 = control-ref of="CODCr检出限"() -> (w45:refnum<vi>)
  n248 = control-ref of="总氮母液浓度"() -> (w50:refnum<vi>)
  n249 = control-ref of="总氮加标体积"() -> (w49:refnum<vi>)
  n250 = control-ref of="COD母液浓度"() -> (w65:refnum<vi>)
  n251 = control-ref of="COD加标体积"() -> (w64:refnum<vi>)
  n252 = control-ref of="总磷母液浓度"() -> (w74:refnum<vi>)
  n253 = control-ref of="总磷加标体积"() -> (w72:refnum<vi>)
  n254 = control-ref of="氨氮母液浓度"() -> (w84:refnum<vi>)
  n255 = control-ref of="氨氮加标体积"() -> (w81:refnum<vi>)
  n256 = control-ref of="CODCr量程"() -> (w46:refnum<vi>)
  n257 = control-ref of="总氮检出限"() -> (w54:refnum<vi>)
  n258 = control-ref of="COD检出限"() -> (w69:refnum<vi>)
  n259 = control-ref of="总磷检出限"() -> (w78:refnum<vi>)
  n260 = control-ref of="氨氮检出限"() -> (w87:refnum<vi>)
  n261 = control-ref of="总氮量程"() -> (w55:refnum<vi>)
  n262 = control-ref of="COD量程"() -> (w70:refnum<vi>)
  n263 = control-ref of="总磷量程"() -> (w79:refnum<vi>)
  n264 = control-ref of="氨氮量程"() -> (w88:refnum<vi>)
  n265 = Obtain Queue(name (unnamed)="质控单元" ("名称（未命名）"), element data type=cluster{"命令":string} {"命令"="启用模块"} ("元素")) -> (queue out=w2:refnum<queue>, error out=w1:errorcluster)  [unwired: 3 in, 1 out]
  n266 = while {
    tunnel: w2 -> [w379]
    tunnel: w1 -> [w378]
    stop <- FALSE stop-if-true
    # "通信入队列"
    n267 = Get Queue Status(queue=w379, error in (no error)=w378) -> (queue out=w376:refnum<queue>, error out=w375:errorcluster, # elements in queue=w377:i32)  [unwired: 1 in, 5 out]
    n268 = Equal To 0?(x=w377) -> (x = 0?=w374:bool)
    n269 = Wait (ms)(milliseconds to wait=u32 1000 ("等待时间（毫秒）")) -> ()  [unwired: 1 out]
    n270 = case shown="真" w374 {
      tunnel: w376 -> [_ w396]
      tunnel: w375 -> [_ w395]
      frame False {
      }
      frame True {
        n271 = local read "氨氮模块"() -> (w394:bool)
        n272 = case shown="真" w394 {
          tunnel: w396 -> [w422 w426]
          tunnel: w395 -> [w421 w425]
          tunnel: [w422 w424] -> w392
          tunnel: [w421 w423] -> w391
          frame False {
          }
          frame True {
            n273 = Enqueue Element(queue=w426, element=cluster{"命令":string} {"命令"="氨氮读取"} ("元素"), error in (no error)=w425) -> (queue out=w424:refnum<queue>, error out=w423:errorcluster)  [unwired: 1 in, 1 out]
          }
        }
        n274 = local read "总磷模块选择"() -> (w393:bool)
        n275 = case shown="真" w393 {
          tunnel: w392 -> [w415 w419]
          tunnel: w391 -> [w414 w418]
          tunnel: [w415 w417] -> w389
          tunnel: [w414 w416] -> w388
          frame False {
          }
          frame True {
            n276 = Enqueue Element(queue=w419, element=cluster{"命令":string} {"命令"="总磷读取"} ("元素"), error in (no error)=w418) -> (queue out=w417:refnum<queue>, error out=w416:errorcluster)  [unwired: 1 in, 1 out]
          }
        }
        n277 = local read "总氮模块选择"() -> (w390:bool)
        n278 = case shown="真" w390 {
          tunnel: w389 -> [w408 w412]
          tunnel: w388 -> [w407 w411]
          tunnel: [w408 w410] -> w386
          tunnel: [w407 w409] -> w385
          frame False {
          }
          frame True {
            n279 = Enqueue Element(queue=w412, element=cluster{"命令":string} {"命令"="总氮读取"} ("元素"), error in (no error)=w411) -> (queue out=w410:refnum<queue>, error out=w409:errorcluster)  [unwired: 1 in, 1 out]
          }
        }
        n280 = local read "CODMn选择"() -> (w387:bool)
        n281 = case shown="真" w387 {
          tunnel: w386 -> [w401 w405]
          tunnel: w385 -> [w400 w404]
          tunnel: [w401 w403] -> w383
          tunnel: [w400 w402] -> w382
          frame False {
          }
          frame True {
            n282 = Enqueue Element(queue=w405, element=cluster{"命令":string} {"命令"="CODMn读取"} ("元素"), error in (no error)=w404) -> (queue out=w403:refnum<queue>, error out=w402:errorcluster)  [unwired: 1 in, 1 out]
          }
        }
        n283 = local read "CODCr选择"() -> (w384:bool)
        n284 = case shown="真" w384 {
          tunnel: w383 -> [_ w398]
          tunnel: w382 -> [_ w397]
          frame False {
          }
          frame True {
            n285 = Enqueue Element(queue=w398, element=cluster{"命令":string} {"命令"="CODCr读取"} ("元素"), error in (no error)=w397) -> ()  [unwired: 1 in, 3 out]
          }
        }
      }
    }
  }
  n286 = property class="VI"(reference=w30) -> ("Name"=w31:string)  [unwired: 1 in, 2 out]
  n287 = Build Array(w46, w45, w44, w43, w42, w41, w40, w39) -> (w38:refnum<vi>[])
  n288 = Build Array(w55, w54, w53, w52, w51, w50, w49, w48) -> (w47:refnum<vi>[])
  n289 = Build Array(w70, w69, w68, w67, w66, w65, w64, w63) -> (w62:refnum<vi>[])
  n290 = Build Array(w79, w78, w77, w76, w75, w74, w72, w73) -> (w71:refnum<vi>[])
  n291 = Build Array(w88, w87, w86, w82, w85, w84, w81, w80) -> (w83:refnum<vi>[])
  n292 = property class="VI"(reference=w17) -> ("Name"=w16:string)  [unwired: 1 in, 2 out]
  n293 = Obtain Notifier(name (unnamed)="采配水Process" ("名称（未命名）"), notification data type=FALSE) -> (notifier out=w59:refnum<notifier>)  [unwired: 2 in, 2 out]
  n294 = Obtain Queue(name (unnamed)="采配水" ("名称（未命名）"), element data type=cluster{"命令":string, "数据":variant} {"命令"="", "数据"=variant}) -> (queue out=w56:refnum<queue>)  [unwired: 3 in, 2 out]
  n295 = Obtain Queue(name (unnamed)="质控单元" ("名称（未命名）"), element data type=cluster{"命令":string} {"命令"="启用模块"} ("元素")) -> (queue out=w27:refnum<queue>, error out=w26:errorcluster)  [unwired: 3 in, 1 out]
  n296 = control-ref of="CODCr加标后水样浓度"() -> (w5:refnum<vi>)
  n297 = property class="VI"(reference=w25) -> ("Name"=w24:string)  [unwired: 1 in, 2 out]
  n298 = control-ref of="总氮加标后水样浓度"() -> (w9:refnum<vi>)
  n299 = control-ref of="COD加标后水样浓度"() -> (w6:refnum<vi>)
  n300 = control-ref of="氨氮加标后水样浓度"() -> (w8:refnum<vi>)
  n301 = control-ref of="总磷加标后水样浓度"() -> (w7:refnum<vi>)
  n302 = Open VI Reference(type specifier VI Refnum (for type only)=refnum<vi> refnum, vi path=w31, options=128 ("选项")) -> (vi reference=w33:refnum<vi>, error out=w35:errorcluster)  [unwired: 3 in]
  n303 = Open VI Reference(type specifier VI Refnum (for type only)=refnum<vi> refnum, vi path=w16, options=128 ("选项")) -> (vi reference=w14:refnum<vi>, error out=w12:errorcluster)  [unwired: 3 in]
  n304 = while {
    tunnel: w83 -> [w436]
    tunnel: w71 -> [w435]
    tunnel: w62 -> [w430]
    tunnel: w59 -> [w434]
    tunnel: w56 -> [w433]
    tunnel: w47 -> [w432]
    tunnel: w38 -> [w431]
    tunnel: w27 -> [w429]
    tunnel: w26 -> [w428]
    stop <- FALSE stop-if-true
    # "氨氮站号是1，总磷站号是2，总氮站号3，CODMn站号是4，CODCr站号是5"
    n305 = event shown="[16] \"柱塞泵调试\": 值改变" {
      selector: _ -> [_ _ _ _ _ _ _ _ _ _ _ _ _ _ _ _ _ _ _ _ _ _ _ _ _]
      dyn-events: _ -> [_ _ _ _ _ _ _ _ _ _ _ _ _ _ _ _ _ _ _ _ _ _ _ _ _]
      timeout: _ -> [_ _ _ _ _ _ _ _ _ _ _ _ _ _ _ _ _ _ _ _ _ _ _ _ _]
      tunnel: w436 -> [_ _ _ _ _ _ _ _ _ _ w537 _ _ _ _ _ _ _ _ _ _ _ _ _ _]
      tunnel: w435 -> [_ _ _ _ _ _ _ _ _ _ _ w551 _ _ _ _ _ _ _ _ _ _ _ _ _]
      tunnel: w430 -> [_ _ _ _ _ _ _ _ _ _ _ _ _ w589 _ _ _ _ _ _ _ _ _ _ _]
      tunnel: w434 -> [_ _ _ _ _ _ _ _ _ _ _ _ _ _ _ _ _ _ _ w675 _ w742 w764 _ _]
      tunnel: w433 -> [_ _ _ _ _ _ _ _ _ _ _ _ _ _ _ _ _ _ _ _ _ _ w761 _ _]
      tunnel: w432 -> [_ _ _ _ _ _ _ _ _ _ _ _ w569 _ _ _ _ _ _ _ _ _ _ _ _]
      tunnel: w431 -> [_ _ _ _ _ _ _ _ _ _ _ _ _ _ w607 _ _ _ _ _ _ _ _ _ _]
      tunnel: w429 -> [_ _ _ _ _ _ _ _ _ _ _ _ _ _ _ _ _ w631 w665 _ _ _ _ _ _]
      tunnel: w428 -> [_ _ _ _ _ _ _ _ _ _ _ _ _ _ _ _ _ w630 w664 _ _ _ _ _ _]
      event Timeout {
        n306 = event-data() -> ()  [unwired: 1 in, 3 out]
      }
      event "氨氮量程", "氨氮检出限", "氨氮加标前水样浓度", "氨氮加标水杯定容体积", "氨氮母液浓度", "氨氮加标后水样浓度": Mouse Down {
        n307 = event-data() -> ("CtlRef"=w441:refnum<vi>)  [unwired: 1 in, 7 out]
        n308 = property class="DigNum (严格)"(reference=w441) -> (reference out=w439:refnum<vi>, "Value"=w440:dbl)  [unwired: 1 in, 1 out]
        n309 = call "数字键盘.vi"("OldNumber"=w440) -> ("NewNumber"=w438:sgl)
        n310 = property class="DigNum (严格)"(reference=w439, "Val(Sgnl)"=w438) -> ()  [unwired: 1 in, 2 out]
      }
      event "总磷母液浓度", "总磷加标水杯定容体积", "总磷加标后水样浓度", "总磷加标前水样浓度", "总磷检出限", "总磷量程": Mouse Down {
        n311 = event-data() -> ("CtlRef"=w445:refnum<vi>)  [unwired: 1 in, 7 out]
        n312 = property class="DigNum (严格)"(reference=w445) -> (reference out=w443:refnum<vi>, "Value"=w444:dbl)  [unwired: 1 in, 1 out]
        n313 = call "数字键盘.vi"("OldNumber"=w444) -> ("NewNumber"=w442:sgl)
        n314 = property class="DigNum (严格)"(reference=w443, "Val(Sgnl)"=w442) -> ()  [unwired: 1 in, 2 out]
      }
      event "总氮母液浓度", "总氮加标水杯定容体积", "总氮加标后水样浓度", "总氮加标前水样浓度", "总氮检出限", "总氮量程": Mouse Down {
        n315 = event-data() -> ("CtlRef"=w449:refnum<vi>)  [unwired: 1 in, 7 out]
        n316 = property class="DigNum (严格)"(reference=w449) -> (reference out=w447:refnum<vi>, "Value"=w448:dbl)  [unwired: 1 in, 1 out]
        n317 = call "数字键盘.vi"("OldNumber"=w448) -> ("NewNumber"=w446:sgl)
        n318 = property class="DigNum (严格)"(reference=w447, "Val(Sgnl)"=w446) -> ()  [unwired: 1 in, 2 out]
      }
      event "COD母液浓度", "COD加标水杯定容体积", "COD加标后水样浓度", "COD加标前水样浓度", "COD检出限", "COD量程": Mouse Down {
        n319 = event-data() -> ("CtlRef"=w453:refnum<vi>)  [unwired: 1 in, 7 out]
        n320 = property class="DigNum (严格)"(reference=w453) -> (reference out=w451:refnum<vi>, "Value"=w452:dbl)  [unwired: 1 in, 1 out]
        n321 = call "数字键盘.vi"("OldNumber"=w452) -> ("NewNumber"=w450:sgl)
        n322 = property class="DigNum (严格)"(reference=w451, "Val(Sgnl)"=w450) -> ()  [unwired: 1 in, 2 out]
      }
      event "CODCr检出限", "CODCr量程", "CODCr加标前水样浓度", "CODCr加标后水样浓度", "CODCr加标水杯定容体积", "CODCr母液浓度": Mouse Down {
        n323 = event-data() -> ("CtlRef"=w454:refnum<vi>)  [unwired: 1 in, 7 out]
        n324 = property class="DigNum (严格)"(reference=w454) -> (reference out=w456:refnum<vi>, "Value"=w457:dbl)  [unwired: 1 in, 1 out]
        n325 = call "数字键盘.vi"("OldNumber"=w457) -> ("NewNumber"=w455:sgl)
        n326 = property class="DigNum (严格)"(reference=w456, "Val(Sgnl)"=w455) -> ()  [unwired: 1 in, 2 out]
      }
      event "背隙补偿步数", "背隙补偿步数 2", "背隙补偿步数 3": Mouse Down {
        n327 = event-data() -> ("CtlRef"=w461:refnum<vi>)  [unwired: 1 in, 7 out]
        n328 = property class="DigNum (严格)"(reference=w461) -> (reference out=w460:refnum<vi>, "Value"=w459:i32)  [unwired: 1 in, 1 out]
        n329 = call "数字键盘.vi"("OldNumber"=w459) -> ("NewNumber"=w458:sgl)
        n330 = property class="DigNum (严格)"(reference=w460, "Val(Sgnl)"=w458) -> ()  [unwired: 1 in, 2 out]
      }
      event "背隙补偿步数", "背隙补偿步数 2", "背隙补偿步数 3": Value Change {
        w470 = "质控背隙补偿" ("section")
        n331 = event-data() -> ()  [unwired: 1 in, 6 out]
        n332 = call <vilib>:"Application Directory.vi"() -> ("Application Directory"=w477:path)
        n333 = Build Path(base path=w477, name or relative path="data\\Set.ini" ("名称或相对路径")) -> (appended path=w475:path)
        n334 = call <vilib>:"Open Config Data.vi"("configuration file path"=w475) -> ("error out"=w473:errorcluster, "refnum"=w474:T3)  [unwired: 8 in, 1 out]
        n335 = call-poly <vilib>:"Write Key.vi"("section"=w470, "error in (no error)"=w473, "value"="背隙补偿步数", "key"="背隙值1", "refnum"=w474) -> ("error out"=w464:errorcluster, "refnum out"=w467:T3)  [unwired: 4 in, 1 out]
        n336 = call-poly <vilib>:"Write Key.vi"("section"=w470, "error in (no error)"=w464, "value"="背隙补偿步数 2", "key"="背隙值2", "refnum"=w467) -> ("error out"=w465:errorcluster, "refnum out"=w466:T3)  [unwired: 4 in, 1 out]
        n337 = call-poly <vilib>:"Write Key.vi"("section"=w470, "error in (no error)"=w465, "value"="背隙补偿步数 3", "key"="背隙值3", "refnum"=w466) -> ()  [unwired: 4 in, 3 out]
      }
      event "氨氮模块", "总磷模块选择", "CODMn选择", "CODCr选择", "总氮模块选择": Value Change {
        w484 = "质控模块选择" ("section")
        n338 = event-data() -> ()  [unwired: 1 in, 6 out]
        n339 = call <vilib>:"Application Directory.vi"() -> ("Application Directory"=w504:path)
        n340 = Build Path(base path=w504, name or relative path="data\\Set.ini" ("名称或相对路径")) -> (appended path=w502:path)
        n341 = local read "氨氮模块"() -> (w494:bool)
        n342 = call <vilib>:"Open Config Data.vi"("configuration file path"=w502) -> ("error out"=w500:errorcluster, "refnum"=w501:T3)  [unwired: 8 in, 1 out]
        n343 = local read "总磷模块选择"() -> (w493:bool)
        n344 = call-poly <vilib>:"Write Key.vi"("section"=w484, "error in (no error)"=w500, "value"=w494, "key"="模块1" ("section"), "refnum"=w501) -> ("error out"=w498:errorcluster, "refnum out"=w499:T3)  [unwired: 4 in, 1 out]
        n345 = local read "总氮模块选择"() -> (w479:bool)
        n346 = call-poly <vilib>:"Write Key.vi"("section"=w484, "error in (no error)"=w498, "value"=w493, "key"="模块2" ("section"), "refnum"=w499) -> ("error out"=w482:errorcluster, "refnum out"=w483:T3)  [unwired: 4 in, 1 out]
        n347 = local read "CODMn选择"() -> (w492:bool)
        n348 = call-poly <vilib>:"Write Key.vi"("section"=w484, "error in (no error)"=w482, "value"=w479, "key"="模块3" ("section"), "refnum"=w483) -> ("error out"=w480:errorcluster, "refnum out"=w481:T3)  [unwired: 4 in, 1 out]
        n349 = local read "CODCr选择"() -> (w486:bool)
        n350 = call-poly <vilib>:"Write Key.vi"("section"=w484, "error in (no error)"=w480, "value"=w492, "key"="模块4" ("section"), "refnum"=w481) -> ("error out"=w489:errorcluster, "refnum out"=w490:T3)  [unwired: 4 in, 1 out]
        n351 = call-poly <vilib>:"Write Key.vi"("section"=w484, "error in (no error)"=w489, "value"=w486, "key"="模块5" ("section"), "refnum"=w490) -> ("error out"=w487:errorcluster, "refnum out"=w488:T3)  [unwired: 4 in, 1 out]
        n352 = call <vilib>:"Close Config Data.vi"("error in (no error)"=w487, "refnum"=w488) -> ("error out"=w478:errorcluster)  [unwired: 8 in, 1 out]
        n353 = call <vilib>:"Clear Errors.vi"("error in (no error)"=w478) -> ()  [unwired: 5 in, 2 out]
      }
      event "氨氮量程选择", "总氮量程选择", "总磷量程选择", "CODMn量程选择", "CODCr量程选择": Value Change {
        w511 = "质控模块量程选择" ("section")
        n354 = event-data() -> ()  [unwired: 1 in, 6 out]
        n355 = call <vilib>:"Application Directory.vi"() -> ("Application Directory"=w530:path)
        n356 = Build Path(base path=w530, name or relative path="data\\Set.ini" ("名称或相对路径")) -> (appended path=w528:path)
        n357 = local read "氨氮量程选择"() -> (w515:enum32{"H", "L", "AUTO"})
        n358 = call <vilib>:"Open Config Data.vi"("configuration file path"=w528) -> ("error out"=w526:errorcluster, "refnum"=w527:T3)  [unwired: 8 in, 1 out]
        n359 = local read "总氮量程选择"() -> (w514:enum32{"H", "L", "AUTO"})
        n360 = call-poly <vilib>:"Write Key.vi"("section"=w511, "error in (no error)"=w526, "value"=w515, "key"="氨氮" ("section"), "refnum"=w527) -> ("error out"=w524:errorcluster, "refnum out"=w525:T3)  [unwired: 4 in, 1 out]
        n361 = local read "总磷量程选择"() -> (w513:enum32{"H", "L", "AUTO"})
        n362 = call-poly <vilib>:"Write Key.vi"("section"=w511, "error in (no error)"=w524, "value"=w514, "key"="总氮" ("section"), "refnum"=w525) -> ("error out"=w522:errorcluster, "refnum out"=w523:T3)  [unwired: 4 in, 1 out]
        n363 = local read "CODMn量程选择"() -> (w512:enum32{"H", "L", "AUTO"})
        n364 = call-poly <vilib>:"Write Key.vi"("section"=w511, "error in (no error)"=w522, "value"=w513, "key"="总磷" ("section"), "refnum"=w523) -> ("error out"=w517:errorcluster, "refnum out"=w518:T3)  [unwired: 4 in, 1 out]
        n365 = local read "CODCr量程选择"() -> (w505:enum32{"H", "L", "AUTO"})
        n366 = call-poly <vilib>:"Write Key.vi"("section"=w511, "error in (no error)"=w517, "value"=w512, "key"="CODMn" ("section"), "refnum"=w518) -> ("error out"=w507:errorcluster, "refnum out"=w510:T3)  [unwired: 4 in, 1 out]
        n367 = call-poly <vilib>:"Write Key.vi"("section"=w511, "error in (no error)"=w507, "value"=w505, "key"="CODCr" ("section"), "refnum"=w510) -> ("error out"=w508:errorcluster, "refnum out"=w509:T3)  [unwired: 4 in, 1 out]
        n368 = call <vilib>:"Close Config Data.vi"("error in (no error)"=w508, "refnum"=w509) -> ()  [unwired: 8 in, 2 out]
      }
      event "氨氮量程", "氨氮检出限", "氨氮加标前水样浓度", "氨氮母液浓度", "氨氮加标水杯定容体积", "氨氮加标后水样浓度": Value Change {
        n369 = event-data() -> ()  [unwired: 1 in, 6 out]
        n370 = for {
          tunnel: w537 -> [w549] mode=indexing
          tunnel: [w548] -> w546 mode=indexing
          n371 = property class="DigNum (严格)"(reference=w549) -> ("Value"=w548:dbl)  [unwired: 1 in, 2 out]
        }
        n372 = Index Array(array=w546) -> (element #1=w545:dbl, element #2=w544:dbl, element #3=w531:dbl, element #4=w543:dbl, element #5=w542:dbl, element #6=w540:dbl)  [unwired: 6 in]
        n373 = global write "水样浓度全局.vi" "氨氮加标前水样浓度"(w531) -> ()
        n374 = Bundle By Name(cluster=T4 {"量程"=0.0, "检出限"=0.0, "加标前水样浓度"=0.0, "加标后水样浓度"=0.0, "加标水杯定容体积"=0.0, "加标母液浓度"=0.0, "加标体积"=0.0, "加标回收率"=0.0} ("参数"), "量程"=w545, "检出限"=w544, "加标前水样浓度"=w531, "加标后水样浓度"=w543, "加标水杯定容体积"=w542, "加标母液浓度"=w540) -> (w539:T4)
        n375 = call "加标回收率计算.vi"("参数"=w539) -> ("参数 out"=w538:T4)  [unwired: 10 in]
        n376 = call "质控参数保存.vi"("section"="氨氮质控参数", "参数"=w538) -> ()  [unwired: 9 in, 1 out]
        n377 = Unbundle By Name(w538) -> ("加标体积"=w532:dbl, "加标回收率"=w533:dbl)
        n378 = Index Array(array=w537, index #1=6 ("索引")) -> (element #1=w536:refnum<vi>, element #2=w534:refnum<vi>)  [unwired: 1 in]
        n379 = property class="DigNum (严格)"(reference=w536, "Value"=w532) -> ()  [unwired: 1 in, 2 out]
        n380 = property class="DigNum (严格)"(reference=w534, "Value"=w533) -> ()  [unwired: 1 in, 2 out]
      }
      event "总磷母液浓度", "总磷加标水杯定容体积", "总磷加标后水样浓度", "总磷加标前水样浓度", "总磷检出限", "总磷量程": Value Change {
        n381 = event-data() -> ()  [unwired: 1 in, 6 out]
        n382 = for {
          tunnel: w551 -> [w568] mode=indexing
          tunnel: [w567] -> w565 mode=indexing
          n383 = property class="DigNum (严格)"(reference=w568) -> ("Value"=w567:dbl)  [unwired: 1 in, 2 out]
        }
        n384 = Index Array(array=w565) -> (element #1=w564:dbl, element #2=w563:dbl, element #3=w550:dbl, element #4=w562:dbl, element #5=w561:dbl, element #6=w559:dbl)  [unwired: 6 in]
        n385 = global write "水样浓度全局.vi" "总磷加标前水样浓度"(w550) -> ()
        n386 = Bundle By Name(cluster=T4 {"量程"=0.0, "检出限"=0.0, "加标前水样浓度"=0.0, "加标后水样浓度"=0.0, "加标水杯定容体积"=0.0, "加标母液浓度"=0.0, "加标体积"=0.0, "加标回收率"=0.0} ("参数"), "量程"=w564, "检出限"=w563, "加标前水样浓度"=w550, "加标后水样浓度"=w562, "加标水杯定容体积"=w561, "加标母液浓度"=w559) -> (w558:T4)
        n387 = call "加标回收率计算.vi"("参数"=w558) -> ("参数 out"=w557:T4)  [unwired: 10 in]
        n388 = call "质控参数保存.vi"("section"="总磷质控参数", "参数"=w557) -> ()  [unwired: 9 in, 1 out]
        n389 = Unbundle By Name(w557) -> ("加标体积"=w554:dbl, "加标回收率"=w552:dbl)
        n390 = Index Array(array=w551, index #1=6 ("索引")) -> (element #1=w556:refnum<vi>, element #2=w553:refnum<vi>)  [unwired: 1 in]
        n391 = property class="DigNum (严格)"(reference=w556, "Value"=w554) -> ()  [unwired: 1 in, 2 out]
        n392 = property class="DigNum (严格)"(reference=w553, "Value"=w552) -> ()  [unwired: 1 in, 2 out]
      }
      event "总氮量程", "总氮检出限", "总氮加标前水样浓度", "总氮加标后水样浓度", "总氮加标水杯定容体积", "总氮母液浓度": Value Change {
        n393 = event-data() -> ()  [unwired: 1 in, 6 out]
        n394 = for {
          tunnel: w569 -> [w587] mode=indexing
          tunnel: [w586] -> w584 mode=indexing
          n395 = property class="DigNum (严格)"(reference=w587) -> ("Value"=w586:dbl)  [unwired: 1 in, 2 out]
        }
        n396 = Index Array(array=w584) -> (element #1=w583:dbl, element #2=w582:dbl, element #3=w570:dbl, element #4=w581:dbl, element #5=w580:dbl, element #6=w578:dbl)  [unwired: 6 in]
        n397 = global write "水样浓度全局.vi" "总氮加标前水样浓度"(w570) -> ()
        n398 = Bundle By Name(cluster=T4 {"量程"=0.0, "检出限"=0.0, "加标前水样浓度"=0.0, "加标后水样浓度"=0.0, "加标水杯定容体积"=0.0, "加标母液浓度"=0.0, "加标体积"=0.0, "加标回收率"=0.0} ("参数"), "量程"=w583, "检出限"=w582, "加标前水样浓度"=w570, "加标后水样浓度"=w581, "加标水杯定容体积"=w580, "加标母液浓度"=w578) -> (w577:T4)
        n399 = call "加标回收率计算.vi"("参数"=w577) -> ("参数 out"=w576:T4)  [unwired: 10 in]
        n400 = call "质控参数保存.vi"("section"="总氮质控参数", "参数"=w576) -> ()  [unwired: 9 in, 1 out]
        n401 = Unbundle By Name(w576) -> ("加标体积"=w573:dbl, "加标回收率"=w571:dbl)
        n402 = Index Array(array=w569, index #1=6 ("索引")) -> (element #1=w575:refnum<vi>, element #2=w572:refnum<vi>)  [unwired: 1 in]
        n403 = property class="DigNum (严格)"(reference=w575, "Value"=w573) -> ()  [unwired: 1 in, 2 out]
        n404 = property class="DigNum (严格)"(reference=w572, "Value"=w571) -> ()  [unwired: 1 in, 2 out]
      }
      event "COD母液浓度", "COD加标水杯定容体积", "COD加标后水样浓度", "COD加标前水样浓度", "COD检出限", "COD量程": Value Change {
        n405 = event-data() -> ()  [unwired: 1 in, 6 out]
        n406 = for {
          tunnel: w589 -> [w606] mode=indexing
          tunnel: [w605] -> w603 mode=indexing
          n407 = property class="DigNum (严格)"(reference=w606) -> ("Value"=w605:dbl)  [unwired: 1 in, 2 out]
        }
        n408 = Index Array(array=w603) -> (element #1=w602:dbl, element #2=w601:dbl, element #3=w588:dbl, element #4=w600:dbl, element #5=w599:dbl, element #6=w597:dbl)  [unwired: 6 in]
        n409 = global write "水样浓度全局.vi" "COD加标前水样浓度"(w588) -> ()
        n410 = Bundle By Name(cluster=T4 {"量程"=0.0, "检出限"=0.0, "加标前水样浓度"=0.0, "加标后水样浓度"=0.0, "加标水杯定容体积"=0.0, "加标母液浓度"=0.0, "加标体积"=0.0, "加标回收率"=0.0} ("参数"), "量程"=w602, "检出限"=w601, "加标前水样浓度"=w588, "加标后水样浓度"=w600, "加标水杯定容体积"=w599, "加标母液浓度"=w597) -> (w596:T4)
        n411 = call "加标回收率计算.vi"("参数"=w596) -> ("参数 out"=w595:T4)  [unwired: 10 in]
        n412 = call "质控参数保存.vi"("section"="COD质控参数", "参数"=w595) -> ()  [unwired: 9 in, 1 out]
        n413 = Unbundle By Name(w595) -> ("加标体积"=w592:dbl, "加标回收率"=w590:dbl)
        n414 = Index Array(array=w589, index #1=6 ("索引")) -> (element #1=w594:refnum<vi>, element #2=w591:refnum<vi>)  [unwired: 1 in]
        n415 = property class="DigNum (严格)"(reference=w594, "Value"=w592) -> ()  [unwired: 1 in, 2 out]
        n416 = property class="DigNum (严格)"(reference=w591, "Value"=w590) -> ()  [unwired: 1 in, 2 out]
      }
      event "CODCr母液浓度", "CODCr加标水杯定容体积", "CODCr加标前水样浓度", "CODCr检出限", "CODCr量程", "CODCr加标后水样浓度": Value Change {
        n417 = event-data() -> ()  [unwired: 1 in, 6 out]
        n418 = for {
          tunnel: w607 -> [w625] mode=indexing
          tunnel: [w624] -> w622 mode=indexing
          n419 = property class="DigNum (严格)"(reference=w625) -> ("Value"=w624:dbl)  [unwired: 1 in, 2 out]
        }
        n420 = Index Array(array=w622) -> (element #1=w621:dbl, element #2=w620:dbl, element #3=w608:dbl, element #4=w619:dbl, element #5=w618:dbl, element #6=w616:dbl)  [unwired: 6 in]
        n421 = global write "水样浓度全局.vi" "CODCr加标前水样浓度"(w608) -> ()
        n422 = Bundle By Name(cluster=T4 {"量程"=0.0, "检出限"=0.0, "加标前水样浓度"=0.0, "加标后水样浓度"=0.0, "加标水杯定容体积"=0.0, "加标母液浓度"=0.0, "加标体积"=0.0, "加标回收率"=0.0} ("参数"), "量程"=w621, "检出限"=w620, "加标前水样浓度"=w608, "加标后水样浓度"=w619, "加标水杯定容体积"=w618, "加标母液浓度"=w616) -> (w615:T4)
        n423 = call "加标回收率计算.vi"("参数"=w615) -> ("参数 out"=w614:T4)  [unwired: 10 in]
        n424 = call "质控参数保存.vi"("section"="CODCr质控参数", "参数"=w614) -> ()  [unwired: 9 in, 1 out]
        n425 = Unbundle By Name(w614) -> ("加标体积"=w611:dbl, "加标回收率"=w609:dbl)
        n426 = Index Array(array=w607, index #1=6 ("索引")) -> (element #1=w613:refnum<vi>, element #2=w610:refnum<vi>)  [unwired: 1 in]
        n427 = property class="DigNum (严格)"(reference=w613, "Value"=w611) -> ()  [unwired: 1 in, 2 out]
        n428 = property class="DigNum (严格)"(reference=w610, "Value"=w609) -> ()  [unwired: 1 in, 2 out]
      }
      event "手动调试": Value Change {
        n429 = event-data() -> ()  [unwired: 1 in, 6 out]
        n430 = call "手动调试界面.vi"() -> ()  [unwired: 16 in]
      }
      event "柱塞泵调试": Value Change {
        n431 = event-data() -> ()  [unwired: 1 in, 6 out]
        n432 = call "柱塞泵调试界面.vi"() -> ()  [unwired: 16 in]
      }
      event "打开串口": Value Change {
        n433 = event-data() -> ()  [unwired: 1 in, 6 out]
        n434 = global read "断电保存全局.vi" "MB通信方式选择"() -> (w626:enum16{"串口", "TCP"})
        n435 = global read "断电保存全局.vi" "VISA Resource"() -> (w627:refnum<visa-resource-name>)
        n436 = global read "断电保存全局.vi" "PORT"() -> (w628:string)
        n437 = global read "断电保存全局.vi" "IP"() -> (w629:string)
        n438 = call "串口配置.vi"("PORT"=w628, "IP"=w629, "MB通信方式选择"=w626, "请选择串口:"=w627) -> ("PORT 2"=w633:string, "IP 2"=w634:string, "确认 2"=w636:bool, "VISA资源名称 2"=w635:refnum<visa-resource-name>, "MB通信方式选择 2"=w632:enum16{"串口", "TCP"})  [unwired: 3 in]
        n439 = case shown="真" w636 {
          tunnel: w635 -> [_ w642]
          tunnel: w631 -> [_ w641]
          tunnel: w634 -> [_ w640]
          tunnel: w633 -> [_ w639]
          tunnel: w632 -> [_ w638]
          tunnel: w630 -> [_ w637]
          frame False {
          }
          frame True {
            n440 = flat-sequence {
              tunnel: w642 -> [w646]
              tunnel: w641 -> [w648]
              tunnel: w640 -> [w645]
              tunnel: w639 -> [w644]
              tunnel: w638 -> [w643]
              tunnel: w637 -> [w647]
              frame #0 {
                n441 = global write "断电保存全局.vi" "IP"(w645) -> ()
                n442 = global write "断电保存全局.vi" "PORT"(w644) -> ()
                n443 = global write "断电保存全局.vi" "VISA Resource"(w646) -> ()
                n444 = global write "断电保存全局.vi" "MB通信方式选择"(w643) -> ()
                n445 = Enqueue Element(queue=w648, element=cluster{"命令":string} {"命令"="启用模块"} ("元素"), error in (no error)=w647) -> ()  [unwired: 1 in, 3 out]
              }
              frame #1 {
                n446 = call <vilib>:"Application Directory.vi"() -> ("Application Directory"=w663:path)
                n447 = Build Path(base path=w663, name or relative path="data\\sys.ini" ("名称或相对路径")) -> (appended path=w661:path)
                n448 = call <vilib>:"Open Config Data.vi"("configuration file path"=w661) -> ("error out"=w657:errorcluster, "refnum"=w660:T3)  [unwired: 8 in, 1 out]
                n449 = vi-ref "质控单元.lvlib:断电保存全局.vi"() -> (w659:refnum<vi>)
                n450 = call <userlib>:"Write Panel to INI__ogtk.vi"("error in (no error)"=w657, "VI ref"=w659, "refnum"=w660) -> ("error out"=w656:errorcluster, "refnum out"=w658:T3)  [unwired: 7 in]
                n451 = call <vilib>:"Close Config Data.vi"("error in (no error)"=w656, "refnum"=w658) -> ("error out"=w651:errorcluster, "file path"=w650:path)  [unwired: 8 in]
                n452 = Open/Create/Replace File(file path (use dialog)=w650, error in=w651) -> (refnum out=w654:refnum<file>, error out=w655:errorcluster)  [unwired: 4 in, 1 out]
                n453 = Flush File(refnum=w654, error in=w655) -> (refnum out=w653:refnum<file>, error out=w652:errorcluster)
                n454 = Close File(refnum=w653, error in=w652) -> ()  [unwired: 2 out]
              }
            }
          }
        }
      }
      event "释放串口": Value Change {
        n455 = event-data() -> ()  [unwired: 1 in, 6 out]
        n456 = Two Button Dialog(message="确认是否释放串口，释放串口将导致通信失败！" ("消息")) -> (T button?=w666:bool)  [unwired: 2 in]
        n457 = case shown="真" w666 {
          tunnel: w665 -> [_ w669]
          tunnel: w664 -> [_ w668]
          frame False {
          }
          frame True {
            n458 = Bundle By Name(cluster=cluster{"命令":string} {"命令"=""} ("元素"), "命令"="停用模块" ("名称（未命名）")) -> (w670:cluster{"命令":string})
            n459 = Enqueue Element(queue=w669, element=w670, error in (no error)=w668) -> ()  [unwired: 1 in, 3 out]
          }
        }
      }
      event "加标回收": Value Change {
        n460 = event-data() -> ()  [unwired: 1 in, 6 out]
        n461 = Send Notification(notification=FALSE ("通知"), notifier=w675) -> ()  [unwired: 1 in, 2 out]
        n462 = call "质控启动流程对话框.vi"() -> ("确定启动"=w673:bool, "启动模块"=w678:T9, "直接启动"=w676:bool, "常规启动"=w677:bool)  [unwired: 8 in]
        n463 = case shown="真" w673 {
          tunnel: w678 -> [_ w687]
          tunnel: w677 -> [_ w686]
          tunnel: w676 -> [_ w685]
          frame False {
          }
          frame True {
            n464 = Bundle By Name(cluster=T6 {"是否启用仪器"=FALSE, "CODMn"={"启动测量模式"={"测量模式"=enum."水样测量"}, "确定按钮"=FALSE}, "启动模块"={"氨氮"=FALSE, "总磷"=FALSE, "总氮"=FALSE, "CODMn"=FALSE, "CODCr"=FALSE}, "常规启动"=FALSE, "直接启动"=FALSE} ("参数"), "是否启用仪器"=TRUE, "启动模块"=w687, "常规启动"=w686, "直接启动"=w685) -> (w679:T6)
            n465 = vi-ref "质控单元.lvlib:一体站流程质控自动启动.vi"() -> (w682:refnum<vi>)
            n466 = property class="VI"(reference=w682) -> ("Name"=w683:string, "Exec.State"=w681:T10)  [unwired: 1 in, 2 out]
            n467 = case shown="\"Idle\"" w681 {
              tunnel: w683 -> [_ w698 _ _]
              tunnel: w679 -> [_ w688 _ _]
              frame "Bad", Default {
              }
              frame "Idle" {
                n468 = Open VI Reference(type specifier VI Refnum (for type only)=refnum<vi> refnum ("类型说明符VI引用句柄（仅用于类型）"), vi path=w698, options=128 ("选项")) -> (vi reference=w699:refnum<vi>, error out=w695:errorcluster)  [unwired: 3 in]
                n469 = call-by-ref "开始异步调用"(reference=w699, error in=w695, "CODMn量程切换"="CODMn量程选择", "总磷量程切换"="总磷量程选择", "总氮量程切换"="总氮量程选择", "氨氮量程切换"="氨氮量程选择", "参数"=w688) -> (reference out=w697:refnum<vi>, error out=w696:errorcluster)  [unwired: 7 in]
                n470 = Close Reference(reference=w697, error in (no error)=w696) -> ()  [unwired: 1 out]
              }
              frame "Run top level" {
              }
              frame "Running" {
                n471 = One Button Dialog(message="流程已启动，无需重复启动！" ("消息")) -> ()  [unwired: 1 in, 1 out]
              }
            }
          }
        }
      }
      event "报警清除": Value Change {
        w701 = u16 259 ("starting address")
        w707 = FALSE ("氨氮中断报警")
        n472 = event-data() -> ()  [unwired: 1 in, 6 out]
        n473 = global write "质控中断报警全局.vi" "氨氮中断报警"(w707) -> ()
        n474 = global write "质控中断报警全局.vi" "CODMn中断报警"(w707) -> ()
        n475 = global write "质控中断报警全局.vi" "总氮中断报警"(w707) -> ()
        n476 = global write "质控中断报警全局.vi" "总磷中断报警"(w707) -> ()
        n477 = global write "质控中断报警全局.vi" "CODCr中断报警"(w707) -> ()
        n478 = local read "氨氮模块"() -> (w711:bool)
        n479 = case shown="真" w711 {
          tunnel: [errorcluster {"status"=FALSE, "code"=0, "source"=""} ("error out") w736] -> w708
          tunnel: w701 -> [_ w735]
          frame False {
          }
          frame True {
            n480 = call "单个写入.vi"("value"=u16 0, "address"=w735, "Slave ID"=u8 1) -> ("error out"=w736:errorcluster)  [unwired: 8 in]
          }
        }
        n481 = local read "总磷模块选择"() -> (w710:bool)
        n482 = case shown="真" w710 {
          tunnel: w708 -> [w728 w731]
          tunnel: [w728 w730] -> w703
          tunnel: w701 -> [_ w729]
          frame False {
          }
          frame True {
            n483 = call "单个写入.vi"("Error in"=w731, "value"=u16 0, "address"=w729, "Slave ID"=u8 2) -> ("error out"=w730:errorcluster)  [unwired: 7 in]
          }
        }
        n484 = local read "总氮模块选择"() -> (w704:bool)
        n485 = case shown="真" w704 {
          tunnel: w703 -> [w712 w715]
          tunnel: [w712 w714] -> w702
          tunnel: w701 -> [_ w713]
          frame False {
          }
          frame True {
            n486 = call "单个写入.vi"("Error in"=w715, "value"=u16 0, "address"=w713, "Slave ID"=u8 3) -> ("error out"=w714:errorcluster)  [unwired: 7 in]
          }
        }
        n487 = local read "CODMn选择"() -> (w709:bool)
        n488 = case shown="真" w709 {
          tunnel: w702 -> [w722 w725]
          tunnel: [w722 w724] -> w705
          tunnel: w701 -> [_ w723]
          frame False {
          }
          frame True {
            n489 = call "单个写入.vi"("Error in"=w725, "value"=u16 0, "address"=w723, "Slave ID"=u8 4) -> ("error out"=w724:errorcluster)  [unwired: 7 in]
          }
        }
        n490 = local read "CODCr选择"() -> (w706:bool)
        n491 = case shown="真" w706 {
          tunnel: w705 -> [_ w719]
          tunnel: w701 -> [_ w718]
          frame False {
          }
          frame True {
            n492 = call "单个写入.vi"("Error in"=w719, "value"=u16 0, "address"=w718, "Slave ID"=u8 5) -> ()  [unwired: 7 in, 1 out]
          }
        }
      }
      event "平行样测试": Value Change {
        n493 = event-data() -> ()  [unwired: 1 in, 6 out]
        n494 = Cancel Notification(0:w742) -> ()  [unwired: 1 in, 3 out]
        n495 = call "平行样启动流程对话框.vi"() -> ("启动模块"=w741:T11, "常规启动"=w739:bool, "确定启动"=w740:bool)  [unwired: 9 in]
        n496 = case shown="真" w740 {
          tunnel: w741 -> [_ w749]
          tunnel: w739 -> [_ w744]
          frame False {
          }
          frame True {
            n497 = Bundle By Name(cluster=T7 {"参数启用"={"CODMn"=FALSE, "总磷"=FALSE, "总氮"=FALSE, "氨氮"=FALSE, "CODcr"=FALSE}, "采配水是否启动"=FALSE} ("参数"), "参数启用"=w749, "采配水是否启动"=w744) -> (w743:T7)
            n498 = vi-ref "质控单元.lvlib:一体站流程平行样自动启动.vi"() -> (w747:refnum<vi>)
            n499 = property class="VI"(reference=w747) -> ("Name"=w748:string, "Exec.State"=w746:T10)  [unwired: 1 in, 2 out]
            n500 = case shown="\"Idle\"" w746 {
              tunnel: w748 -> [_ w756]
              tunnel: w743 -> [_ w750]
              frame "Bad", Default {
              }
              frame "Idle" {
                n501 = Open VI Reference(type specifier VI Refnum (for type only)=refnum<vi> refnum ("类型说明符VI引用句柄（仅用于类型）"), vi path=w756, options=128 ("选项")) -> (vi reference=w757:refnum<vi>, error out=w755:errorcluster)  [unwired: 3 in]
                n502 = call-by-ref "开始异步调用"(reference=w757, error in=w755, "参数"=w750) -> (reference out=w752:refnum<vi>, error out=w751:errorcluster)  [unwired: 11 in]
                n503 = Close Reference(reference=w752, error in (no error)=w751) -> ()  [unwired: 1 out]
              }
            }
          }
        }
      }
      event "停止测量": Value Change {
        w758 = TRUE ("氨氮")
        # "停止采配水、氨氮、总磷总氮、COD、质控"
        n504 = event-data() -> ()  [unwired: 1 in, 6 out]
        n505 = Send Notification(notification=TRUE ("通知"), notifier=w764) -> ()  [unwired: 1 in, 2 out]
        n506 = Enqueue Element At Opposite End(queue=w761, element=T8 {"命令"="单个写入", {"starting address"=300, "holding register value"=2}} ("元素")) -> ()  [unwired: 2 in, 3 out]
        n507 = call "质控启动参数选择对话框.vi"("CODCr"=w758, "CODMn"=w758, "总氮"=w758, "总磷"=w758, "氨氮"=w758) -> ("确定启动"=w759:bool, "启动模块"=w760:T9)  [unwired: 4 in, 1 out]
        n508 = case shown="真" w759 {
          tunnel: w760 -> [_ w770]
          frame False {
          }
          frame True {
            n509 = Unbundle By Name(w770) -> ("氨氮"=w768:bool, "总磷"=w766:bool, "总氮"=w765:bool, "CODMn"=w769:bool, "CODCr"=w767:bool)
            n510 = case shown="真" w766 {
              frame False {
              }
              frame True {
                n511 = call "加标仪器启动命令 (子VI).vi"("启动命令"=enum16{"启动水样流程", "启动加标流程", "排液", "停止"}."停止", "仪器"=enum16{"", "氨氮", "总磷", "总氮", "CODMn", "CODCr"}."总磷") -> ()  [unwired: 9 in, 1 out]
                n512 = Obtain Queue(name (unnamed)="TP" ("名称（未命名）"), element data type=cluster{"命令":string, "data":variant} {"命令"="", "data"=variant}) -> (queue out=w796:refnum<queue>)  [unwired: 3 in, 2 out]
                n513 = Obtain Notifier(name (unnamed)="TP" ("名称（未命名）"), notification data type=FALSE) -> (notifier out=w792:refnum<notifier>)  [unwired: 2 in, 2 out]
                n514 = Send Notification(notification=TRUE ("通知"), notifier=w792) -> ()  [unwired: 1 in, 2 out]
                n515 = Enqueue Element(queue=w796, element=cluster{"命令":string, "data":variant} {"命令"="启动", "data"=variant(cluster{"站号":u16, "控制命令输出":u16[]} {"站号"=1, "控制命令输出"=[2816]})} ("元素")) -> ()  [unwired: 2 in, 3 out]
              }
            }
            n516 = case shown="真" w765 {
              frame False {
              }
              frame True {
                n517 = call "加标仪器启动命令 (子VI).vi"("启动命令"=enum16{"启动水样流程", "启动加标流程", "排液", "停止"}."停止", "仪器"=enum16{"", "氨氮", "总磷", "总氮", "CODMn", "CODCr"}."总氮") -> ()  [unwired: 9 in, 1 out]
                n518 = Obtain Queue(name (unnamed)="TN" ("名称（未命名）"), element data type=cluster{"命令":string, "data":variant} {"命令"="", "data"=variant}) -> (queue out=w780:refnum<queue>)  [unwired: 3 in, 2 out]
                n519 = Obtain Notifier(name (unnamed)="TN" ("名称（未命名）"), notification data type=FALSE) -> (notifier out=w776:refnum<notifier>)  [unwired: 2 in, 2 out]
                n520 = Send Notification(notification=TRUE ("通知"), notifier=w776) -> ()  [unwired: 1 in, 2 out]
                n521 = Enqueue Element(queue=w780, element=cluster{"命令":string, "data":variant} {"命令"="启动", "data"=variant(cluster{"站号":u16, "控制命令输出":u16[]} {"站号"=1, "控制命令输出"=[2816]})} ("元素")) -> ()  [unwired: 2 in, 3 out]
              }
            }
            n522 = case shown="真" w769 {
              frame False {
              }
              frame True {
                n523 = call "CODMn停止命令 (子VI).vi"() -> ()  [unwired: 12 in]
                n524 = Obtain Notifier(name (unnamed)="CODMn" ("名称（未命名）"), notification data type=FALSE) -> (notifier out=w809:refnum<notifier>)  [unwired: 2 in, 2 out]
                n525 = Send Notification(notification=TRUE ("通知"), notifier=w809) -> ()  [unwired: 1 in, 2 out]
                n526 = call "加标仪器启动命令 (子VI).vi"("启动命令"=enum16{"启动水样流程", "启动加标流程", "排液", "停止"}."停止", "仪器"=enum16{"", "氨氮", "总磷", "总氮", "CODMn", "CODCr"}."CODMn") -> ()  [unwired: 9 in, 1 out]
              }
            }
            n527 = case shown="真" w767 {
              frame False {
              }
              frame True {
                n528 = call "CODCr停止命令 (子VI).vi"() -> ()  [unwired: 12 in]
                n529 = Obtain Notifier(name (unnamed)="CODCr" ("名称（未命名）"), notification data type=FALSE) -> (notifier out=w783:refnum<notifier>)  [unwired: 2 in, 2 out]
                n530 = Send Notification(notification=TRUE ("通知"), notifier=w783) -> ()  [unwired: 1 in, 2 out]
                n531 = call "加标仪器启动命令 (子VI).vi"("启动命令"=enum16{"启动水样流程", "启动加标流程", "排液", "停止"}."停止", "仪器"=enum16{"", "氨氮", "总磷", "总氮", "CODMn", "CODCr"}."CODCr") -> ()  [unwired: 9 in, 1 out]
              }
            }
            n532 = case shown="真" w768 {
              frame False {
              }
              frame True {
                n533 = call "加标仪器启动命令 (子VI).vi"("启动命令"=enum16{"启动水样流程", "启动加标流程", "排液", "停止"}."停止", "仪器"=enum16{"", "氨氮", "总磷", "总氮", "CODMn", "CODCr"}."氨氮") -> ()  [unwired: 9 in, 1 out]
                n534 = Obtain Notifier(name (unnamed)="NH3N" ("名称（未命名）"), notification data type=FALSE) -> (notifier out=w802:refnum<notifier>)  [unwired: 2 in, 2 out]
                n535 = Obtain Queue(name (unnamed)="NH3N" ("名称（未命名）"), element data type=cluster{"命令":string, "data":variant} {"命令"="", "data"=variant}) -> (queue out=w806:refnum<queue>)  [unwired: 3 in, 2 out]
                n536 = Send Notification(notification=TRUE ("通知"), notifier=w802) -> ()  [unwired: 1 in, 2 out]
                n537 = Enqueue Element(queue=w806, element=cluster{"命令":string, "data":variant} {"命令"="启动", "data"=variant(cluster{"站号":u16, "控制命令输出":u16[]} {"站号"=1, "控制命令输出"=[2816]})} ("元素")) -> ()  [unwired: 2 in, 3 out]
              }
            }
          }
        }
      }
      event "查看": Value Change {
        n538 = event-data() -> ()  [unwired: 1 in, 6 out]
        n539 = property on="窗格" class="Pane"("Origin"=T2 {"Horizontal"=0, "Vertical"=640} ("原点")) -> ()  [unwired: 2 in, 2 out]
      }
      event "返回": Value Change {
        n540 = event-data() -> ()  [unwired: 1 in, 6 out]
        n541 = property on="窗格" class="Pane"("Origin"=T2 {"Horizontal"=0, "Vertical"=0} ("原点")) -> ()  [unwired: 2 in, 2 out]
      }
    }
  }
  n542 = call-by-ref "?"(reference=w33, error in=w35) -> (reference out=w37:refnum<vi>, error out=w36:errorcluster)  [unwired: 12 in]
  n543 = Open VI Reference(type specifier VI Refnum (for type only)=refnum<vi> refnum, vi path=w24, options=128 ("选项")) -> (vi reference=w22:refnum<vi>, error out=w20:errorcluster)  [unwired: 3 in]
  n544 = call-by-ref "?"(reference=w22, error in=w20) -> (reference out=w18:refnum<vi>, error out=w19:errorcluster)  [unwired: 12 in]
  n545 = Close Reference(reference=w37, error in (no error)=w36) -> ()  [unwired: 1 out]
  n546 = call-by-ref "?"(reference=w14, error in=w12, "CODMn"=w6, "总磷"=w7, "CODCr"=w5, "氨氮"=w8, "总氮"=w9) -> (reference out=w10:refnum<vi>, error out=w11:errorcluster)  [unwired: 7 in]
  n547 = Close Reference(reference=w18, error in (no error)=w19) -> ()  [unwired: 1 out]
  n548 = Close Reference(reference=w10, error in (no error)=w11) -> ()  [unwired: 1 out]
